vi "MegaAwesome_11_16_12a_OriginDis_JW.vi"() -> ()   [LabVIEW 2011]
uses:
  data/MegaAwesome_States.ctl
  <vilib>/Utility/inputDevices.llb/keyboardAcquire.vi
  <vilib>/Utility/file.llb/Read From Spreadsheet File (string).vi
  <vilib>/Utility/file.llb/Write To Spreadsheet File (string).vi
panel:
  out "Save Next?":bool
  out "Image Center X":i32
  in  "Disable Flag":bool
  out "Index":string
  in  "Slider Min":dbl=5.0
  in  "Slider Max":dbl=5.0
  out "Opj X Axis":string
  out "X Axis Display Type":string
  in  "Index-Sat":dbl=5.0
  in  "Index-Lin":dbl=5.0
  in  "IndexLog-Lin":dbl=5.0
  in  "IndexLog-Sat":dbl=5.0 caption="Num Pts"
  out "Lin Id-Log Used":dbl[](array[numeric])
  out "Lin-Vg Array-Log Used":dbl[](array[numeric])
  out "Save Array":string[][](array[string])
  out "Folder Index":i32 caption="Length"
  out "Sat Id-Used":dbl[](array[numeric])
  out "Sat Vg Array-Used":dbl[](array[numeric])
  out "Vg Array-Log-Used":dbl[](array[numeric])
  out "Sat Id-Log-Used":dbl[](array[numeric])
  out "Lin Id-Used":dbl[](array[numeric])
  out "Lin-Vg Array-Used":dbl[](array[numeric])
  out "Lin Vd":dbl
  out "Recorded Prop":T1
  out "Current State":T2
  in  "Main Tab Control":T3(tab)
  in  "Transfer File":path
  out "Transfer Folder":path
  in  "Transport\nFolder":path caption="Transport Folder"
  out "Transport\nFile":path caption="Transport File"
  in  "Image Folder":path
  out "Image File":path
  out "Fabrication Prop":T4
  out "Distances":i32[](array[numeric])
  in  "Zoom":i32(slide)=-3 scale=-5.0..5.0
  in  "Magnification":i32(ring) items=["5x", "10x", "20x", "50x", "80x"]
  in  "Undo Button":bool
  in  "Remove Button":bool
  in  "Transfer Plots":T5(tab)=enum."Saturation"
  in  "Lin-Trans Slider":dbl(slide) step=1.0 scale=-40.0..40.0 scale format="%#_1p"
  out "Sqrt-Lin":cluster{dbl[], dbl[]}[](graph)
  in  "Sat-Trans Slider":dbl(slide) step=1.0 scale=-40.0..40.0 scale format="%#_1p"
  out "Sqrt-Sat":cluster{dbl[], dbl[]}[](graph)
  out "Raw- Lin":cluster{dbl[], dbl[]}[](graph)
  out "Raw- Sat":cluster{dbl[], dbl[]}[](graph)
  in  "Log Plots":enum32{"Linear", "Saturation", "Transport"}(tab)=enum."Saturation"
  in  "Lin-Log Slider":dbl(slide) step=1.0 scale=-40.0..40.0 scale format="%#_1p"
  out "Lin-Log":cluster{dbl[], dbl[]}[](graph)
  in  "Sat-Log Slider":dbl(slide) step=1.0 scale=-40.0..40.0 scale format="%#_1p"
  out "Sat-Log":cluster{dbl[], dbl[]}[](graph)
  out "Transport":cluster{ext[], ext[]}[](graph)
  out "Transport Name:":string
  in  "Manual Controls":T6
  in  "File Controls":T7
  out "Date Recorded":string="Date Recorded" caption="Measured"
  out "Data Name:":string
  out "Image Name":string
  out "Date Created":string caption="Fabricated"
  in  "Comments:":string
  out "Rec: Length":dbl caption="Length"
  out "Rec: Width":dbl caption="Width"
  out "Rec: Dielectric (d)":dbl caption="Dielectric (d)" format="%#_3g"
  in  "New: Dielectric":dbl
  in  "New: Length":dbl
  in  "New: Width":dbl
  out "Rec: Temp":dbl caption="Sample Temp" format="%.1f"
  in  "New: Temp":dbl format="%.1f"
  out "Image Out":T8(plugin-control)
  in  "Num Pts":i32=5
  in  "Num Pts Log":i32=5 caption="Num Pts"
  out "Recorded Values Cluster":T9
  out "Calculated Values Cluster":T9 caption="Recorded Values Cluster"
  out "Re-Calculated Values Cluster":T9 caption="Recorded Values Cluster"
  in  "Independant Variable:":string(combo)="Length (um):"
  out "Image Preview":T8(plugin-control)
  out "Total Width":i32
  in  "Index Array":i32(ring) caption="Index" items=["4C", "4C", "4C", "4C", "4C", "4C", "4C", "4C", "4C", "4C", "4C", "4C", "4C", "4C", "4C", "4C", "4C", "4C", "4C", "4C", "4C", "4C", "4C", "4C", "4C", "4C", "4C", "4C", "4C", "4C", "4C", "4C", "4C", "4C", "4C", "4C", "4C", "4C", "4C"]
  in  "Room Temp":dbl=294.0 caption="Room Temp (K)"
  out "No Image\n File":path=path "\\\\acad1\\physics/Jurchescu-group/JW-PD/Mega Awesome/Image Not Found.png" caption="No Image File"
  out "Origin Project File":path=path "\\\\acad1\\physics/Jurchescu-group/JW-PD/Group Library/Origin Project Files/DeviceData_8_10_12a_JW.opj"
  out "No Transport\n File":path=path "\\\\acad1\\physics/Jurchescu-group/JW-PD/Mega Awesome/No Transport File.txt" caption="No Transport File"
  in  "Transport Style Controls":T10={"Transport Line Size"=1, "Transport Line Color"=16772608} {"Transport Line Size" items=["Extra Small", "Small", "Medium", "Large", "Extra Large"]}
  out "Application Directory":path
  # "1)  Select the Transfer File that you would like to analyze:"
  # "Transfer Location"
  # "2) What else would you like to view during your analysis?"
  # "Transport Location"
  # "Image Location"
  # "Recorded"
  # "Calculated"
  # "Re-Calculated"
  # "Manual"
  # "um"
  # "V"
  # "V"
  # "V"
  # "Default File Choices"
  # "Default Analysis Values"
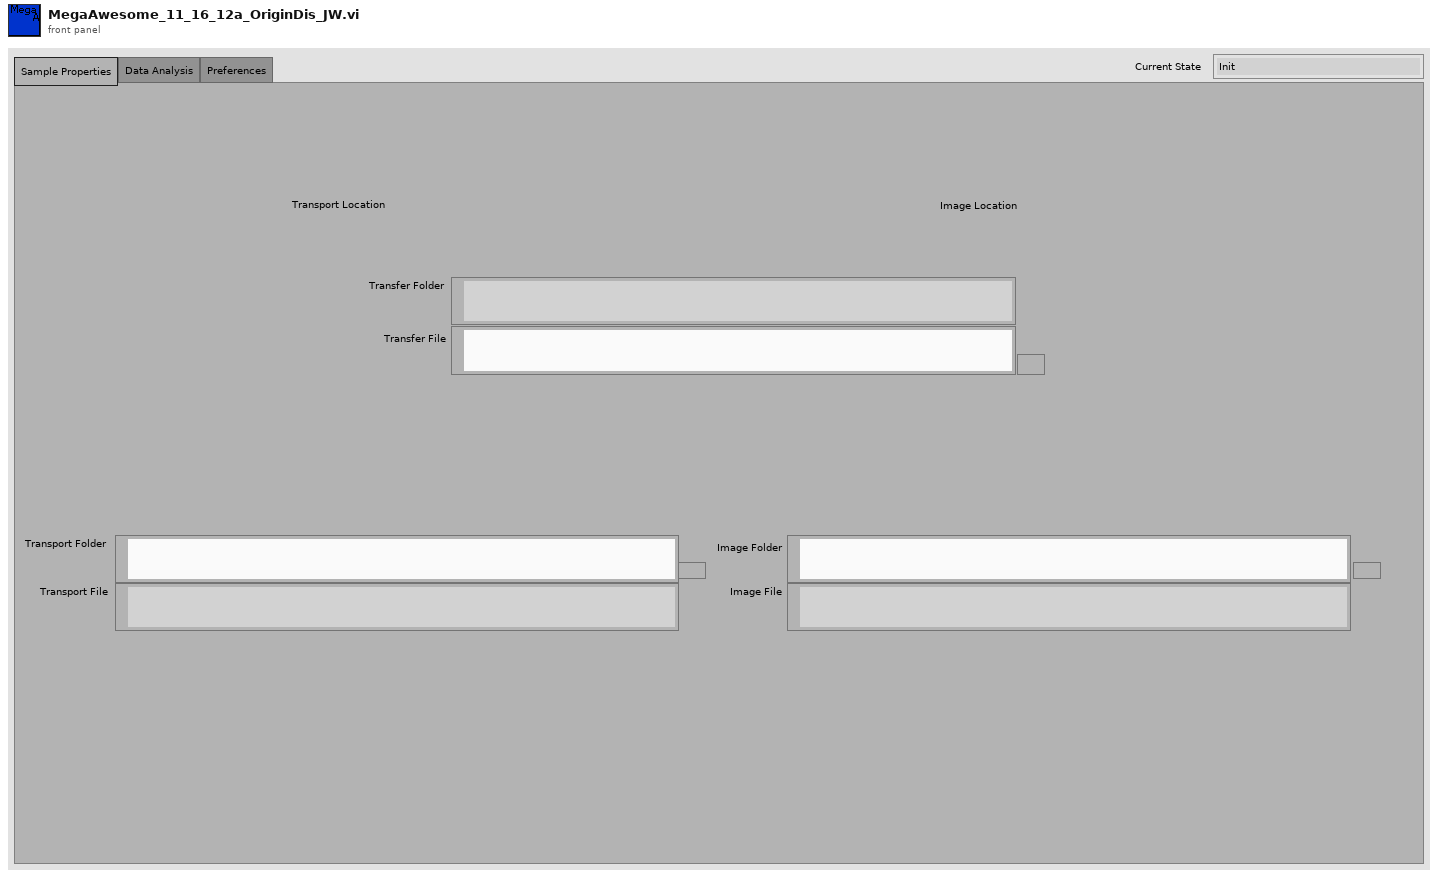
[diagram p1: front panel]
types:
  T1 = cluster{"Date Recorded":string, "Index":string, "Length":dbl, "Width":dbl, "Sample Temp":dbl}
  T2 = typedef "MegaAwesome_States.ctl" = enum16{"Init", "File Missing", "No Event", "Read Data", "Calculated Values", "Re-Calculated Values", "Next File", "Previous File", "Discard File", "Save", "Save Lines", "Export", "Exit"}
  T3 = enum32{"Sample Properties", "Data Analysis", "Preferences"}
  T4 = cluster{"Date Created":string, "Material":string, "Solvent":string, "Concentration":dbl, "Method":string, "Dielectric (nm)":dbl, "Treatment":string, "Comments":string}
  T5 = enum32{"Linear", "Saturation", "Raw-Linear", "Raw-Saturation"}
  T6 = cluster{"Manual-Temp":bool, "Manual-Width":bool, "Manuel-Length":bool, "Manuel-Dielectric":bool, "Manual Comments":bool}
  T7 = cluster{"Previous File":bool, "Discard ":bool, "Save Lines":bool, "Close":bool, "Next File ":bool, "Save":bool, "Save Next":bool, "Export":bool}
  T8 = typedef "IMAQ Image.ctl" = refnum<image>
  T9 = cluster{"Mobility-Sat":dbl, "Moblitity-Lin":dbl, "On/Off":dbl, "Off Current":dbl, "Vt-Sat":dbl, "STS":dbl, "Trap Density-VT":dbl, "Trap Density-STS":dbl}
  T10 = cluster{"Transport Line Size":u16, "Transport Line Color":u32}
  T11 = enum8{"Enabled", "Disabled", "Disabled and Grayed Out"}
  T12 = typedef "LVBoundsTypeDef.ctl" = cluster{"Width":u32, "Height":u32}
  T13 = enum16{"0", "1", "2", "3", "4", "5", "6", "7", "8", "9", "A", "B", "C", "D", "E", "F", "G", "H", "I", "J", "K", "L", "M", "N", "O", "P", "Q", "R", "S", "T", "U", "V", "W", "X", "Y", "Z", "F1", "F2", "F3", "F4", "F5", "F6", "F7", "F8", "F9", "F10", "F11", "F12", "F13", "F14", "F15", "ADD", "BACK", "BACKSLASH", "CAPITAL", "COMMA", "DECIMAL", "DELETE", "DIVIDE", "DOWN", "END", "EQUALS", "ESCAPE", "GRAVE (`)", "HOME", "INSERT", "LBRACKET", "LCONTROL", "LEFT", "L ALT", "LSHIFT", "LWIN", "MINUS", "MULTIPLY", "NEXT", "NUMLOCK", "NUMPAD_0", "NUMPAD_1", "NUMPAD_2", "NUMPAD_3", "NUMPAD_4", "NUMPAD_5", "NUMPAD_6", "NUMPAD_7", "NUMPAD_8", "NUMPAD_9", "PAUSE", "PERIOD", "PRIOR (PG UP)", "RBRACKET", "RCONTROL", "RETURN", "RIGHT", "R ALT", "RSHIFT", "RWIN", "SCROLL", "SEMICOLON", "SLASH", "SPACE", "SUBTRACT", "TAB", "UP", "ENTER (num pad)", "' (quote)"}[]
  T14 = enum16{"0", "1", "2", "3", "4", "5", "6", "7", "8", "9", "A", "B", "C", "D", "E", "F", "G", "H", "I", "J", "K", "L", "M", "N", "O", "P", "Q", "R", "S", "T", "U", "V", "W", "X", "Y", "Z", "F1", "F2", "F3", "F4", "F5", "F6", "F7", "F8", "F9", "F10", "F11", "F12", "F13", "F14", "F15", "ADD", "BACK", "BACKSLASH", "CAPITAL", "COMMA", "DECIMAL", "DELETE", "DIVIDE", "DOWN", "END", "EQUALS", "ESCAPE", "GRAVE (`)", "HOME", "INSERT", "LBRACKET", "LCONTROL", "LEFT", "L ALT", "LSHIFT", "LWIN", "MINUS", "MULTIPLY", "NEXT", "NUMLOCK", "NUMPAD_0", "NUMPAD_1", "NUMPAD_2", "NUMPAD_3", "NUMPAD_4", "NUMPAD_5", "NUMPAD_6", "NUMPAD_7", "NUMPAD_8", "NUMPAD_9", "PAUSE", "PERIOD", "PRIOR (PG UP)", "RBRACKET", "RCONTROL", "RETURN", "RIGHT", "R ALT", "RSHIFT", "RWIN", "SCROLL", "SEMICOLON", "SLASH", "SPACE", "SUBTRACT", "TAB", "UP", "ENTER (num pad)", "' (quote)"}
  T15 = typedef "ROI Descriptor" = cluster{"Global Rectangle":i32[], "Contours":cluster{"ID":enum32{"External", "Internal"}, "Type":u32, "Coordinates":i32[]}[]}
  T16 = cluster{string, sgl, bool, bool, bool, bool, bool, bool, i32}
  T17 = cluster{i32, cluster{string, sgl, bool, bool, bool, bool, bool, bool, i32}, i32, i32}
  T18 = cluster{"Global Rectangle":i32[], "Contours":cluster{"Contour Type":u32, "ROI Type":u32, "Points":i32[]}[]}
  T19 = cluster{"Contour Type":u32, "ROI Type":u32, "Points":i32[]}[]
  T20 = cluster{"[0]":cluster{dbl[], dbl[]}, "[1]":cluster{dbl[], dbl[]}, "[2]":cluster{dbl[], dbl[]}, "[3]":cluster{dbl[], dbl[]}, "[4]":cluster{dbl[], dbl[]}, "[5]":cluster{dbl[], dbl[]}, "[6]":cluster{dbl[], dbl[]}, "[7]":cluster{dbl[], dbl[]}, "[8]":cluster{dbl[], dbl[]}}
  T21 = cluster{i32[], cluster{"Contour Type":u32, "ROI Type":u32, "Points":i32[]}[]}
  T22 = cluster{"Contour Type":u32, "ROI Type":u32, "Points":i32[]}
  T23 = cluster{"Points[0]":i32, "Points[1]":i32, "Points[2]":i32, "Points[3]":i32, "Points[4]":i32, "Points[5]":i32, "Points[6]":i32, "Points[7]":i32, "Points[8]":i32}
  T24 = cluster{"Sat Vg Used":dbl[], "Sat Sqrt(Id) Used ":dbl[], "Lin Vg Used":dbl[], "Lin Sqrt(Id) Used":dbl[], "Index-Lin":dbl, "Index-Sat":dbl}
  T25 = cluster{"Raw Sat":cluster{dbl[], dbl[]}[], "Sqrt Sat":cluster{dbl[], dbl[]}[], "Log Sat":cluster{dbl[], dbl[]}[], "Raw Lin":cluster{dbl[], dbl[]}[], "Sqrt Lin":cluster{dbl[], dbl[]}[], "Log Lin":cluster{dbl[], dbl[]}[]}
  T26 = cluster{"Mobility-Sat":dbl, "Vt-Sat":dbl, "Mobility-Lin":dbl, "Vt-Lin":dbl, "Off I-Sat":dbl, "On/Off I-Sat":dbl}
  T27 = cluster{"Sat Vg Used":dbl[], "Sat Log(Id) Used":dbl[], "Lin Vg Used":dbl[], "Lin Log(Id) Used":dbl[], "STS Index-Sat":dbl, "STS Index-Lin":dbl}
  T28 = cluster{"Independant  Variable Indicator":string, "Parameter String Indicator":string}
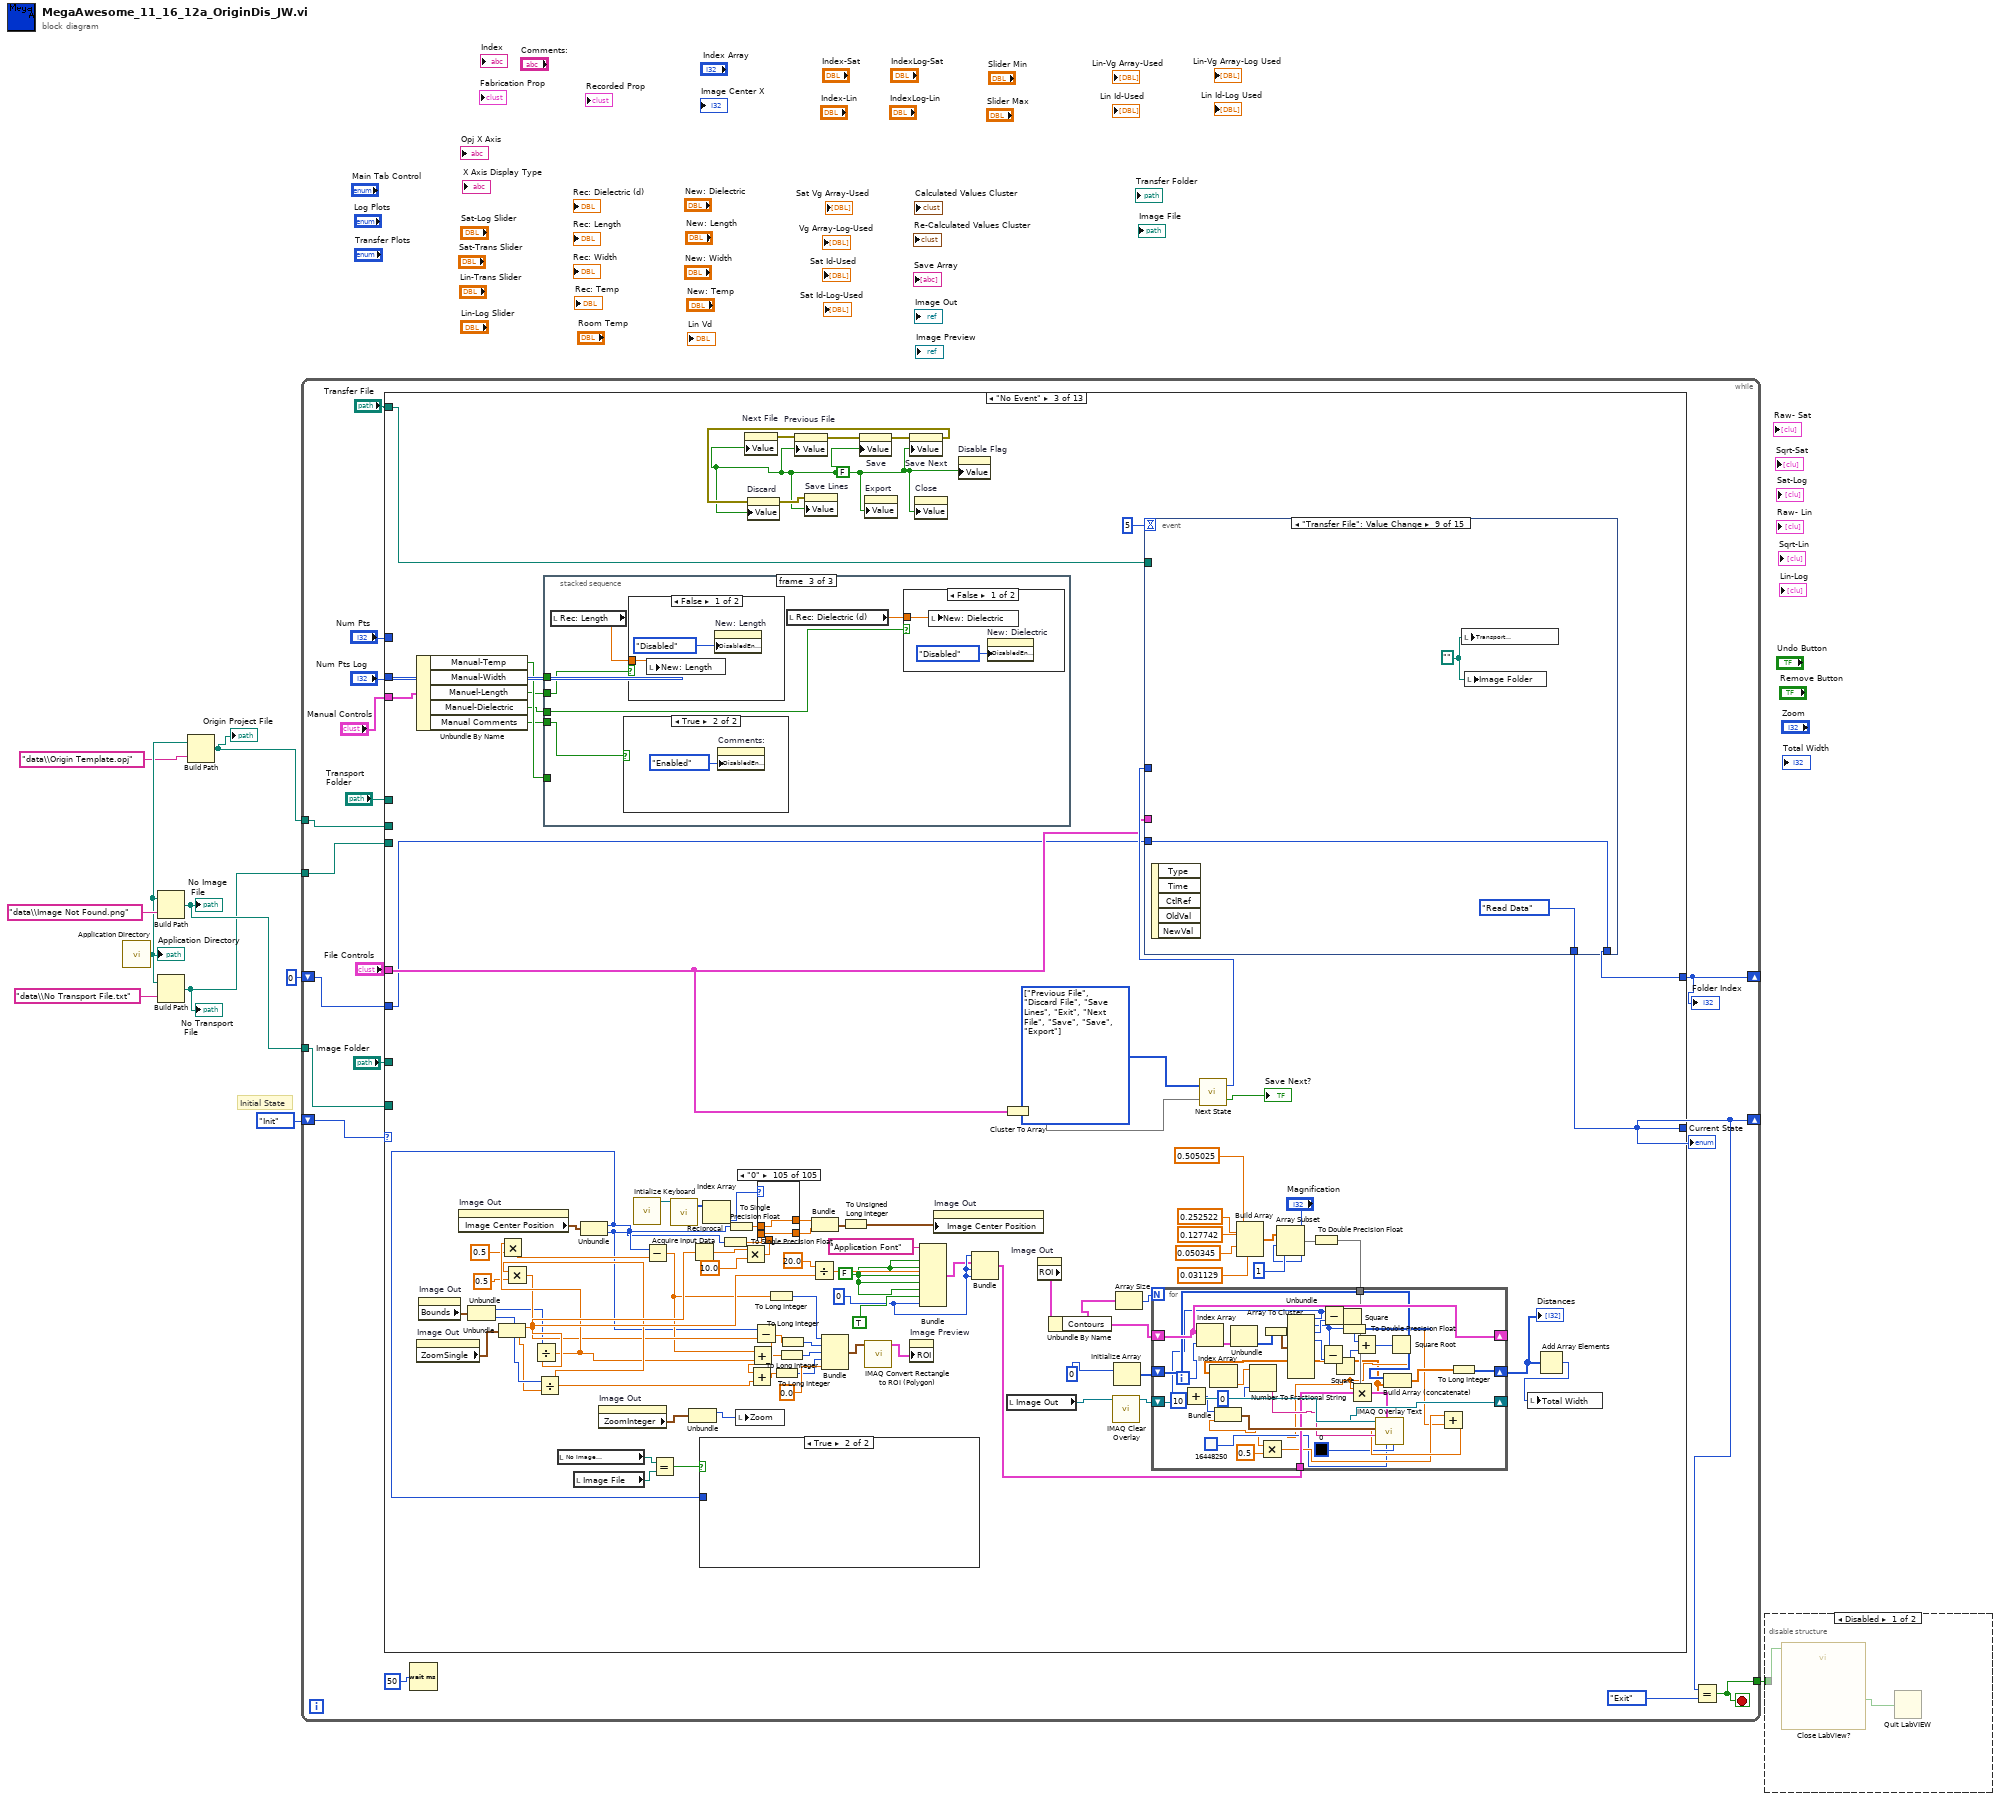
[diagram p0: block diagram]
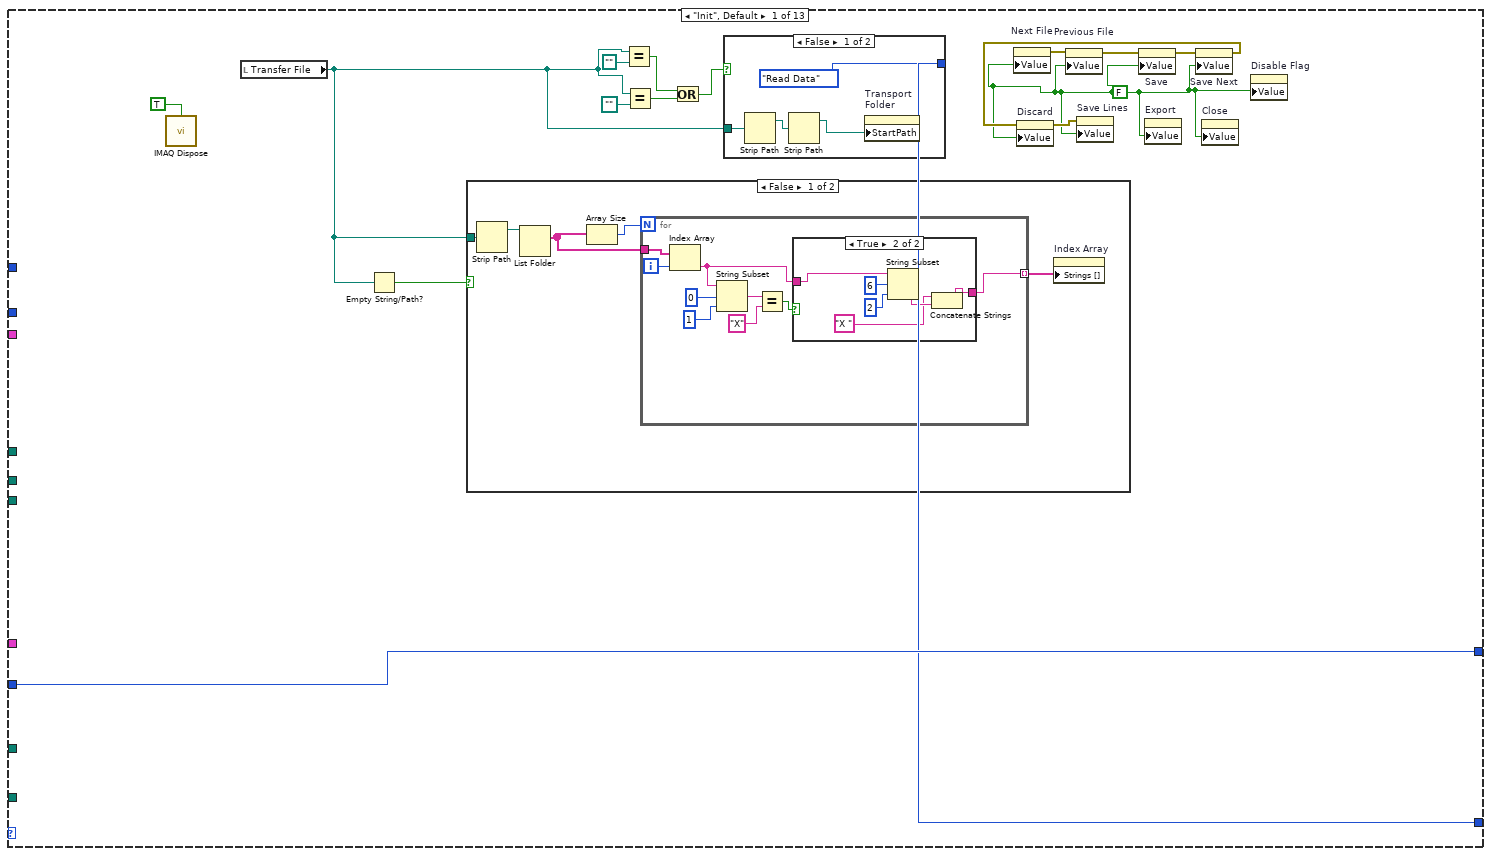
[diagram p3: hidden frame]
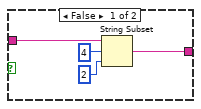
[diagram p4: hidden frame]
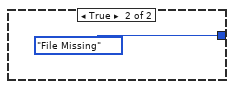
[diagram p6: hidden frame]
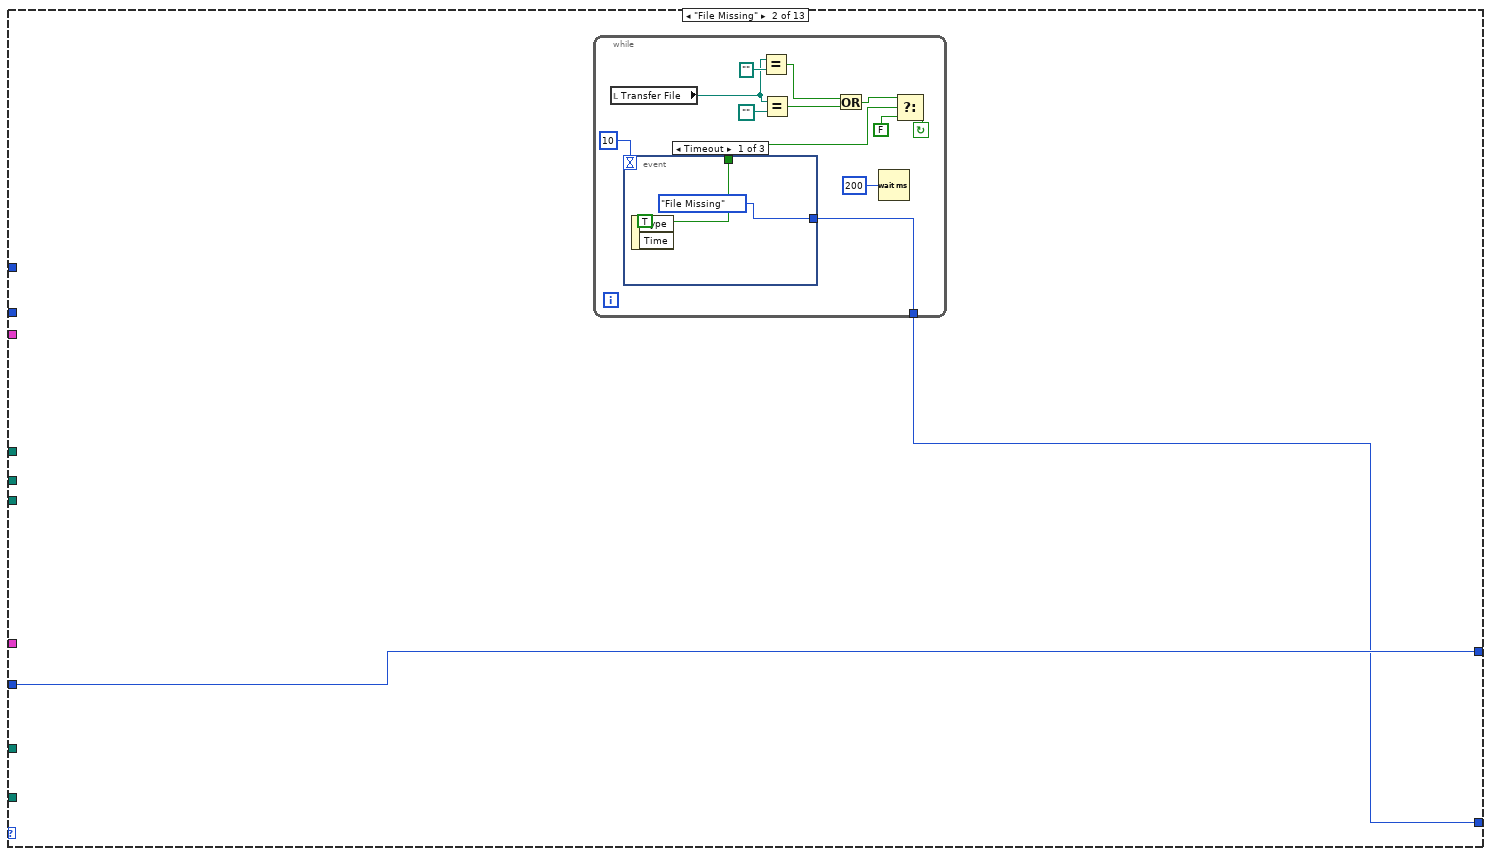
[diagram p7: hidden frame]
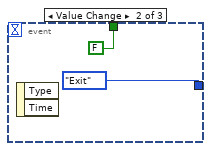
[diagram p8: hidden frame]
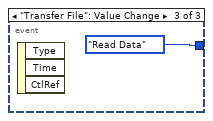
[diagram p9: hidden frame]
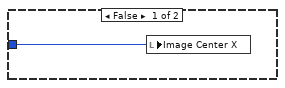
[diagram p10: hidden frame]
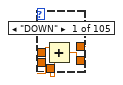
[diagram p11: hidden frame]
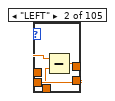
[diagram p12: hidden frame]
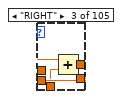
[diagram p13: hidden frame]
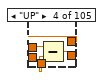
[diagram p14: hidden frame]
diagram:
  # "Initial State"
  n1 = call <vilib>:"Application Directory.vi"() -> ("Application Directory"=w3:path)
  "Application Directory" <- w3
  n2 = Build Path(base path=w3, name or relative path="data\\Image Not Found.png") -> (appended path=w6:path)
  "No Image\n File" <- w6
  n3 = Build Path(base path=w3, name or relative path="data\\No Transport File.txt") -> (appended path=w5:path)
  "No Transport\n File" <- w5
  n4 = Build Path(base path=w3, name or relative path="data\\Origin Template.opj") -> (appended path=w4:path)
  "Origin Project File" <- w4
  n5 = while {
    shift-right: [w11] -> _
    shift-left: MegaAwesome_States."Init" -> [w13]
    shift-right: [w21] -> _
    shift-left: 0 -> [w22]
    tunnel: w6 -> [w18]
    tunnel: w5 -> [w16]
    tunnel: w4 -> [w15]
    tunnel: [w14] -> w1
    stop <- w14 stop-if-true
    n6 = case shown="\"No Event\"" w13 {
      tunnel: [w29 w73 w174 MegaAwesome_States."Calculated Values" MegaAwesome_States."Re-Calculated Values" MegaAwesome_States."No Event" MegaAwesome_States."Read Data" MegaAwesome_States."Read Data" MegaAwesome_States."Init" w828 MegaAwesome_States."Exit" MegaAwesome_States."No Event" MegaAwesome_States."No Event"] -> w11
      tunnel: "Transfer File" -> [_ _ w166 w627 w675 _ w776 w787 w814 w833 _ _ _]
      tunnel: "Num Pts" -> [_ _ _ _ w710 _ _ _ _ _ _ _ _]
      tunnel: "Num Pts Log" -> [_ _ _ _ w709 _ _ _ _ _ _ _ _]
      tunnel: "Image Folder" -> [_ _ _ _ w706 _ _ _ _ _ _ w1340 _]
      tunnel: w18 -> [_ _ _ _ w705 _ _ _ _ _ _ _ _]
      tunnel: [w38 w74 w167 w632 w704 w736 w762 w785 w810 w834 w1326 w1350 w1356] -> w21
      tunnel: w22 -> [w38 w74 w108 w630 w704 w736 w763 w786 _ w834 w1326 w1350 w1356]
      tunnel: "Manual Controls" -> [_ _ w176 _ _ _ _ _ _ w832 _ _ _]
      tunnel: "File Controls" -> [_ _ w164 _ _ _ _ _ _ _ _ _ _]
      tunnel: "Transport\nFolder" -> [_ _ _ _ w671 _ _ _ _ _ _ _ _]
      tunnel: w16 -> [_ _ _ _ w670 _ _ _ _ _ _ _ _]
      tunnel: w15 -> [_ _ _ _ _ _ _ _ _ _ _ _ w1355]
      frame "Init", Default {
        w30 = FALSE
        n7 = call "IMAQ Dispose"("All Images? (No)"=TRUE) -> ()  [unwired: 5 in, 1 out]
        n8 = local read "Transfer File"() -> (w28:path)
        n9 = Empty String/Path?(string/path=w28) -> (empty?=w37:bool)
        n10 = case shown="False" w37 {
          tunnel: w28 -> [w45 _]
          frame False {
            n11 = Strip Path(path=w45) -> (stripped path=w47:path)  [unwired: 1 out]
            n12 = List Folder(path=w47) -> (filenames=w46:string[])  [unwired: 3 in, 3 out]
            n13 = Array Size(array=w46) -> (size(s)=w48:i32)
            n14 = for {
              N: w48 -> [_]
              tunnel: w46 -> [w57]
              tunnel: [w55] -> w44 mode=indexing
              i -> [w56]
              n15 = Index Array(array=w57, index=w56) -> (element=w54:string)
              n16 = String Subset(string=w54, offset (0)=0, length (rest)=1) -> (substring=w51:string)
              n17 = Equal?(x=w51, y="X") -> (x = y?=w50:bool)
              n18 = case shown="True" w50 {
                tunnel: w54 -> [w61 w65]
                tunnel: [w58 w64] -> w55
                frame False {
                  n19 = String Subset(string=w61, offset (0)=4, length (rest)=2) -> (substring=w58:string)
                }
                frame True {
                  n20 = String Subset(string=w65, offset (0)=6, length (rest)=2) -> (substring=w63:string)
                  n21 = Concatenate Strings("X ", w63) -> (w64:string)
                }
              }
            }
            n22 = property on="Index Array" class="Ring (strict)"("Strings []"=w44) -> ()  [unwired: 2 in, 2 out]
          }
          frame True {
          }
        }
        n23 = Equal?(x=w28, y=path "") -> (x = y?=w41:bool)
        n24 = Equal?(x=w28, y=path "") -> (x = y?=w40:bool)
        n25 = Or(x=w41, y=w40) -> (x .or. y?=w43:bool)
        n26 = case shown="False" w43 {
          tunnel: [MegaAwesome_States."Read Data" MegaAwesome_States."File Missing"] -> w29
          tunnel: w28 -> [w70 _]
          frame False {
            n27 = Strip Path(path=w70) -> (stripped path=w69:path)  [unwired: 1 out]
            n28 = Strip Path(path=w69) -> (stripped path=w68:path)  [unwired: 1 out]
            n29 = property on="Transport\nFolder" class="Path"("StartPath"=w68) -> ()  [unwired: 2 in, 2 out]
          }
          frame True {
          }
        }
        n30 = property on="Next File" class="Bool (strict)"("Value"=w30) -> (error out=w35:errorcluster)  [unwired: 2 in, 1 out]
        n31 = property on="Previous File" class="Bool (strict)"(error in=w35, "Value"=w30) -> (error out=w34:errorcluster)  [unwired: 1 in, 1 out]
        n32 = property on="Save" class="Bool (strict)"(error in=w34, "Value"=w30) -> (error out=w33:errorcluster)  [unwired: 1 in, 1 out]
        n33 = property on="Export" class="Bool (strict)"("Value"=w30) -> ()  [unwired: 2 in, 2 out]
        n34 = property on="Save Next" class="Bool (strict)"(error in=w33, "Value"=w30) -> (error out=w32:errorcluster)  [unwired: 1 in, 1 out]
        n35 = property on="Discard" class="Bool (strict)"(error in=w32, "Value"=w30) -> (error out=w31:errorcluster)  [unwired: 1 in, 1 out]
        n36 = property on="Save Lines" class="Bool (strict)"(error in=w31, "Value"=w30) -> ()  [unwired: 1 in, 2 out]
        n37 = property on="Close" class="Bool (strict)"("Value"=w30) -> ()  [unwired: 2 in, 2 out]
        n38 = property on="Disable Flag" class="Bool (strict)"("Value"=w30) -> ()  [unwired: 2 in, 2 out]
      }
      frame "File Missing" {
        n39 = while {
          tunnel: [w81] -> w73
          stop <- w77 continue-if-true
          n40 = local read "Transfer File"() -> (w82:path)
          n41 = event shown="[0] Timeout" {
            selector: _ -> [_ _ _]
            dyn-events: _ -> [_ _ _]
            timeout: 10 -> [_ _ _]
            tunnel: [MegaAwesome_States."File Missing" MegaAwesome_States."Exit" MegaAwesome_States."Read Data"] -> w81
            tunnel: [TRUE FALSE _] -> w80
            event Timeout {
              n42 = event-data() -> ()  [unwired: 1 in, 2 out]
            }
            event "File Controls.Close": Value Change {
              n43 = event-data() -> ()  [unwired: 1 in, 2 out]
            }
            event "Transfer File": Value Change {
              n44 = event-data() -> ()  [unwired: 1 in, 3 out]
            }
          }
          n45 = Equal?(x=w82, y=path "") -> (x = y?=w84:bool)
          n46 = Equal?(x=w82, y=path "") -> (x = y?=w85:bool)
          n47 = Or(x=w84, y=w85) -> (x .or. y?=w79:bool)
          n48 = Wait (ms)(milliseconds to wait=u32 200) -> ()  [unwired: 1 out]
          n49 = Select(t=w79, s=w80, f=FALSE) -> (s? t:f=w77:bool)
        }
      }
      frame "No Event" {
        w155 = FALSE
        w157 = 0
        w165 = FALSE
        w183 = T2[] [enum."Previous File", enum."Discard File", enum."Save Lines", enum."Exit", enum."Next File", enum."Save", enum."Save", enum."Export"] items=["Init", "File Missing", "No Event", "Read Data", "Calculated Values", "Re-Calculated Values", "Next File", "Previous File", "Discard File", "Save", "Save Lines", "Export", "Exit"]
        n50 = Unbundle By Name(w176) -> ("Manual-Temp"=w181:bool, "Manual-Width"=w180:bool, "Manuel-Length"=w179:bool, "Manuel-Dielectric"=w178:bool, "Manual Comments"=w177:bool)
        n51 = property on="Image Out" class="ImageControl"() -> ("ZoomSingle"=w144:cluster{"X":sgl, "Y":sgl})  [unwired: 2 in, 2 out]
        n52 = property on="Image Out" class="ImageControl"() -> ("Bounds"=w143:T12)  [unwired: 2 in, 2 out]
        n53 = property on="Image Out" class="ImageControl"() -> ("Image Center Position"=w140:cluster{"X":u32, "Y":u32})  [unwired: 2 in, 2 out]
        n54 = Unbundle(w143) -> ("Width"=w146:u32, "Height"=w147:u32)
        n55 = Unbundle(w144) -> ("X"=w161:sgl, "Y"=w145:sgl)
        n56 = Divide(x=w146, y=w161) -> (x/y=w152:sgl)
        n57 = Multiply(x=w152, y=sgl 0.5) -> (x*y=w150:sgl)
        n58 = Divide(x=w147, y=w145) -> (x/y=w153:sgl)
        n59 = Multiply(x=w153, y=sgl 0.5) -> (x*y=w151:sgl)
        n60 = stacked-sequence {
          tunnel: w181 -> [w585 _ _]
          tunnel: w180 -> [_ w599 _]
          tunnel: w179 -> [_ _ w612]
          tunnel: w178 -> [_ _ w610]
          tunnel: w177 -> [_ _ w609]
          frame #0 {
            n61 = local read "Rec: Temp"() -> (w584:dbl)
            n62 = case shown="True" w585 {
              tunnel: w584 -> [w590 _]
              frame False {
                n63 = local read "Rec: Temp"() -> (w588:dbl)
                n64 = property on="New: Temp" class="DigNum (strict)"("DisabledEnum"=T11."Disabled" ("Disabled")) -> ()  [unwired: 2 in, 2 out]
                n65 = Equal To 0?(x=w588) -> (x = 0?=w589:bool)
                n66 = local write "New: Temp"(w590) -> ()
                n67 = case shown="True" w589 {
                  tunnel: [w591 w592] -> w586
                  tunnel: w588 -> [w591 _]
                  frame False {
                  }
                  frame True {
                    n68 = local read "Room Temp"() -> (w592:dbl)
                  }
                }
                n69 = local write "Rec: Temp"(w586) -> ()
                n70 = local write "New: Temp"(w586) -> ()
              }
              frame True {
                n71 = property on="New: Temp" class="DigNum (strict)"("DisabledEnum"=T11."Enabled" ("Disabled")) -> ()  [unwired: 2 in, 2 out]
              }
            }
          }
          frame #1 {
            n72 = local read "New: Width"() -> (w600:dbl)
            n73 = local read "Total Width"() -> (w596:i32)
            n74 = case shown="False" w599 {
              frame False {
                n75 = property on="New: Width" class="DigNum (strict)"("DisabledEnum"=T11."Disabled" ("Disabled")) -> ()  [unwired: 2 in, 2 out]
              }
              frame True {
                n76 = property on="New: Width" class="DigNum (strict)"("DisabledEnum"=T11."Enabled" ("Disabled")) -> ()  [unwired: 2 in, 2 out]
              }
            }
            n77 = Not(x=w599) -> (.not. x?=w594:bool)
            n78 = Not Equal?(x=w596, y=w600) -> (x != y?=w595:bool)
            n79 = Equal To 0?(x=w596) -> (x = 0?=w598:bool)
            n80 = And(x=w594, y=w598) -> (x .and. y?=w597:bool)
            n81 = case shown="False" w597 {
              tunnel: w596 -> [w604 _]
              tunnel: w595 -> [w603 _]
              tunnel: w594 -> [w602 _]
              frame False {
                n82 = And(x=w602, y=w603) -> (x .and. y?=w601:bool)
                n83 = case shown="True" w601 {
                  tunnel: w604 -> [_ w605]
                  frame False {
                  }
                  frame True {
                    n84 = property on="New: Width" class="DigNum (strict)"("Val(Sgnl)"=w605) -> ()  [unwired: 2 in, 2 out]
                  }
                }
              }
              frame True {
                n85 = local read "Rec: Width"() -> (w606:dbl)
                n86 = local write "New: Width"(w606) -> ()
              }
            }
          }
          frame #2 {
            n87 = local read "Rec: Length"() -> (w613:dbl)
            n88 = case shown="True" w609 {
              frame False {
                n89 = property on="Comments:" class="Str"("DisabledEnum"=T11."Disabled" ("Disabled")) -> ()  [unwired: 2 in, 2 out]
              }
              frame True {
                n90 = property on="Comments:" class="Str"("DisabledEnum"=T11."Enabled" ("Disabled")) -> ()  [unwired: 2 in, 2 out]
              }
            }
            n91 = case shown="False" w612 {
              tunnel: w613 -> [w620 _]
              frame False {
                n92 = local write "New: Length"(w620) -> ()
                n93 = property on="New: Length" class="DigNum (strict)"("DisabledEnum"=T11."Disabled" ("Disabled")) -> ()  [unwired: 2 in, 2 out]
              }
              frame True {
                n94 = property on="New: Length" class="DigNum (strict)"("DisabledEnum"=T11."Enabled" ("Disabled")) -> ()  [unwired: 2 in, 2 out]
              }
            }
            n95 = local read "Rec: Dielectric (d)"() -> (w611:dbl)
            n96 = case shown="False" w610 {
              tunnel: w611 -> [w617 _]
              frame False {
                n97 = local write "New: Dielectric"(w617) -> ()
                n98 = property on="New: Dielectric" class="DigNum (strict)"("DisabledEnum"=T11."Disabled" ("Disabled")) -> ()  [unwired: 2 in, 2 out]
              }
              frame True {
                n99 = property on="New: Dielectric" class="DigNum (strict)"("DisabledEnum"=T11."Enabled" ("Disabled")) -> ()  [unwired: 2 in, 2 out]
              }
            }
          }
        }
        n100 = local read "No Image\n File"() -> (w114:path)
        n101 = local read "Image File"() -> (w113:path)
        n102 = Unbundle(w140) -> ("X"=w94:u32, "Y"=w92:u32)
        n103 = property on="Image Out" class="ImageControl"() -> ("ZoomInteger"=w117:cluster{"X":i32, "Y":i32})  [unwired: 2 in, 2 out]
        n104 = call <vilib>:"Intialize Keyboard.vi"() -> ("device ID"=w138:refnum<k1>)  [unwired: 10 in, 1 out]
        n105 = Subtract(x=w94, y=w150) -> (x-y=w102:sgl)
        n106 = Equal?(x=w114, y=w113) -> (x = y?=w112:bool)
        n107 = call-poly <vilib>:"Acquire Input Data.vi"("device ID"=w138) -> ("keys pressed"=w139:T13)  [unwired: 16 in, 2 out]
        n108 = Unbundle(w117) -> ("X"=w116:i32)  [unwired: 1 out]
        n109 = Reciprocal(x=w161) -> (1/x=w162:sgl)
        n110 = case shown="True" w112 {
          tunnel: w94 -> [w184 _]
          frame False {
            n111 = local write "Image Center X"(w184) -> ()
          }
          frame True {
          }
        }
        n112 = Index Array(array=w139) -> (element=w96:T14)  [unwired: 1 in]
        n113 = To Single Precision Float(number=w92) -> (single precision float=w93:sgl)
        n114 = To Single Precision Float(number=w94) -> (single precision float=w95:sgl)
        n115 = local write "Zoom"(w116) -> ()
        n116 = Multiply(x=w162, y=sgl 10.0) -> (x*y=w160:sgl)
        n117 = property on="Next File" class="Bool (strict)"("Value"=w165) -> (error out=w172:errorcluster)  [unwired: 2 in, 1 out]
        n118 = Add(x=w102, y=w152) -> (x+y=w100:sgl)
        n119 = Subtract(x=w92, y=w151) -> (x-y=w104:sgl)
        n120 = Add(x=w104, y=w153) -> (x+y=w98:sgl)
        n121 = case shown="\"0\"" w96 {
          tunnel: w95 -> [w221 w227 w231 w233 w237 w239 w241 w243 w245 w247 w249 w251 w253 w255 w257 w259 w261 w263 w265 w267 w269 w271 w273 w275 w277 w279 w281 w283 w285 w287 w289 w291 w293 w295 w297 w299 w301 w303 w305 w307 w309 w311 w313 w315 w317 w319 w321 w323 w325 w327 w329 w331 w333 w335 w337 w339 w341 w343 w345 w347 w349 w351 w353 w355 w357 w359 w361 w363 w365 w367 w369 w371 w373 w375 w377 w379 w381 w383 w385 w387 w389 w391 w393 w395 w397 w399 w401 w403 w405 w407 w409 w411 w413 w415 w417 w419 w421 w423 w425 w427 w429 w431 w433 w435 w437]
          tunnel: [w221 w226 w230 w233 w237 w239 w241 w243 w245 w247 w249 w251 w253 w255 w257 w259 w261 w263 w265 w267 w269 w271 w273 w275 w277 w279 w281 w283 w285 w287 w289 w291 w293 w295 w297 w299 w301 w303 w305 w307 w309 w311 w313 w315 w317 w319 w321 w323 w325 w327 w329 w331 w333 w335 w337 w339 w341 w343 w345 w347 w349 w351 w353 w355 w357 w359 w361 w363 w365 w367 w369 w371 w373 w375 w377 w379 w381 w383 w385 w387 w389 w391 w393 w395 w397 w399 w401 w403 w405 w407 w409 w411 w413 w415 w417 w419 w421 w423 w425 w427 w429 w431 w433 w435 w437] -> w136
          tunnel: w93 -> [w223 w225 w229 w235 w236 w238 w240 w242 w244 w246 w248 w250 w252 w254 w256 w258 w260 w262 w264 w266 w268 w270 w272 w274 w276 w278 w280 w282 w284 w286 w288 w290 w292 w294 w296 w298 w300 w302 w304 w306 w308 w310 w312 w314 w316 w318 w320 w322 w324 w326 w328 w330 w332 w334 w336 w338 w340 w342 w344 w346 w348 w350 w352 w354 w356 w358 w360 w362 w364 w366 w368 w370 w372 w374 w376 w378 w380 w382 w384 w386 w388 w390 w392 w394 w396 w398 w400 w402 w404 w406 w408 w410 w412 w414 w416 w418 w420 w422 w424 w426 w428 w430 w432 w434 w436]
          tunnel: [w222 w225 w229 w234 w236 w238 w240 w242 w244 w246 w248 w250 w252 w254 w256 w258 w260 w262 w264 w266 w268 w270 w272 w274 w276 w278 w280 w282 w284 w286 w288 w290 w292 w294 w296 w298 w300 w302 w304 w306 w308 w310 w312 w314 w316 w318 w320 w322 w324 w326 w328 w330 w332 w334 w336 w338 w340 w342 w344 w346 w348 w350 w352 w354 w356 w358 w360 w362 w364 w366 w368 w370 w372 w374 w376 w378 w380 w382 w384 w386 w388 w390 w392 w394 w396 w398 w400 w402 w404 w406 w408 w410 w412 w414 w416 w418 w420 w422 w424 w426 w428 w430 w432 w434 w436] -> w137
          tunnel: w160 -> [w220 w224 w228 w232 _ _ _ _ _ _ _ _ _ _ _ _ _ _ _ _ _ _ _ _ _ _ _ _ _ _ _ _ _ _ _ _ _ _ _ _ _ _ _ _ _ _ _ _ _ _ _ _ _ _ _ _ _ _ _ _ _ _ _ _ _ _ _ _ _ _ _ _ _ _ _ _ _ _ _ _ _ _ _ _ _ _ _ _ _ _ _ _ _ _ _ _ _ _ _ _ _ _ _ _ _]
          frame "DOWN" {
            n122 = Add(x=w223, y=w220) -> (x+y=w222:sgl)
          }
          frame "LEFT" {
            n123 = Subtract(x=w227, y=w224) -> (x-y=w226:sgl)
          }
          frame "RIGHT" {
            n124 = Add(x=w231, y=w228) -> (x+y=w230:sgl)
          }
          frame "UP" {
            n125 = Subtract(x=w235, y=w232) -> (x-y=w234:sgl)
          }
          frame "ENTER (num pad)" {
          }
          frame "' (quote)" {
          }
          frame "END" {
          }
          frame "EQUALS" {
          }
          frame "ESCAPE" {
          }
          frame "GRAVE (`)" {
          }
          frame "HOME" {
          }
          frame "INSERT" {
          }
          frame "LBRACKET" {
          }
          frame "LCONTROL" {
          }
          frame "L ALT" {
          }
          frame "LSHIFT" {
          }
          frame "LWIN" {
          }
          frame "MINUS" {
          }
          frame "MULTIPLY" {
          }
          frame "NEXT" {
          }
          frame "NUMLOCK" {
          }
          frame "NUMPAD_0" {
          }
          frame "NUMPAD_1" {
          }
          frame "NUMPAD_2" {
          }
          frame "NUMPAD_3" {
          }
          frame "NUMPAD_4" {
          }
          frame "NUMPAD_5" {
          }
          frame "NUMPAD_6" {
          }
          frame "NUMPAD_7" {
          }
          frame "NUMPAD_8" {
          }
          frame "NUMPAD_9" {
          }
          frame "PAUSE" {
          }
          frame "PERIOD" {
          }
          frame "PRIOR (PG UP)" {
          }
          frame "RBRACKET" {
          }
          frame "RCONTROL" {
          }
          frame "RETURN" {
          }
          frame "R ALT" {
          }
          frame "RSHIFT" {
          }
          frame "RWIN" {
          }
          frame "SCROLL" {
          }
          frame "SEMICOLON" {
          }
          frame "SLASH" {
          }
          frame "SPACE" {
          }
          frame "SUBTRACT" {
          }
          frame "TAB" {
          }
          frame "DIVIDE" {
          }
          frame "DELETE" {
          }
          frame "DECIMAL" {
          }
          frame "COMMA" {
          }
          frame "CAPITAL" {
          }
          frame "BACKSLASH" {
          }
          frame "BACK" {
          }
          frame "ADD" {
          }
          frame "F15" {
          }
          frame "F14" {
          }
          frame "F13" {
          }
          frame "F12" {
          }
          frame "F11" {
          }
          frame "F10" {
          }
          frame "F9" {
          }
          frame "F8" {
          }
          frame "F7" {
          }
          frame "F6" {
          }
          frame "F5" {
          }
          frame "F4" {
          }
          frame "F3" {
          }
          frame "F2" {
          }
          frame "F1" {
          }
          frame "Z" {
          }
          frame "Y" {
          }
          frame "X" {
          }
          frame "W" {
          }
          frame "V" {
          }
          frame "U" {
          }
          frame "T" {
          }
          frame "S" {
          }
          frame "R" {
          }
          frame "Q" {
          }
          frame "P" {
          }
          frame "O" {
          }
          frame "N" {
          }
          frame "M" {
          }
          frame "L" {
          }
          frame "K" {
          }
          frame "J" {
          }
          frame "I" {
          }
          frame "H" {
          }
          frame "G" {
          }
          frame "F" {
          }
          frame "E" {
          }
          frame "D" {
          }
          frame "C" {
          }
          frame "B" {
          }
          frame "A" {
          }
          frame "9" {
          }
          frame "8" {
          }
          frame "7" {
          }
          frame "6" {
          }
          frame "5" {
          }
          frame "4" {
          }
          frame "3" {
          }
          frame "2" {
          }
          frame "1" {
          }
          frame "0" {
          }
        }
        n126 = To Long Integer(number=w102) -> (32bit integer=w101:i32)
        n127 = To Long Integer(number=w98) -> (32bit integer=w97:i32)
        n128 = To Long Integer(number=w100) -> (32bit integer=w99:i32)
        n129 = To Long Integer(number=w104) -> (32bit integer=w103:i32)
        n130 = property on="Previous File" class="Bool (strict)"(error in=w172, "Value"=w165) -> (error out=w171:errorcluster)  [unwired: 1 in, 1 out]
        n131 = Divide(x=sgl 20.0, y=w161) -> (x/y=w159:sgl)
        n132 = Bundle(w136, w137) -> (w107:cluster{sgl, sgl})  [unwired: 1 in]
        n133 = Bundle(w101, w103, w99, w97, 0.0) -> (w105:cluster{i32, i32, i32, i32, dbl})  [unwired: 1 in]
        n134 = To Unsigned Long Integer(number=w107) -> (unsigned 32bit integer=w106:cluster{u32, u32})
        n135 = property on="Save" class="Bool (strict)"(error in=w171, "Value"=w165) -> (error out=w170:errorcluster)  [unwired: 1 in, 1 out]
        n136 = property on="Export" class="Bool (strict)"("Value"=w165) -> ()  [unwired: 2 in, 2 out]
        n137 = call "IMAQ Convert Rectangle to ROI (Polygon)"("Rectangle"=w105) -> ("ROI Descriptor"=w142:T15)  [unwired: 7 in, 2 out]
        n138 = property on="Save Next" class="Bool (strict)"(error in=w170, "Value"=w165) -> (error out=w169:errorcluster)  [unwired: 1 in, 1 out]
        n139 = property on="Discard" class="Bool (strict)"(error in=w169, "Value"=w165) -> (error out=w168:errorcluster)  [unwired: 1 in, 1 out]
        n140 = property on="Save Lines" class="Bool (strict)"(error in=w168, "Value"=w165) -> ()  [unwired: 1 in, 2 out]
        n141 = property on="Image Preview" class="ImageControl"("ROI"=w142) -> ()  [unwired: 2 in, 2 out]
        n142 = property on="Close" class="Bool (strict)"("Value"=w165) -> ()  [unwired: 2 in, 2 out]
        n143 = Bundle("Application Font", w159, w155, w155, w155, w155, w155, TRUE, w157) -> (w154:T16)  [unwired: 1 in]
        n144 = property on="Image Out" class="ImageControl"("Image Center Position"=w106) -> ()  [unwired: 2 in, 2 out]
        n145 = property on="Disable Flag" class="Bool (strict)"("Value"=w165) -> ()  [unwired: 2 in, 2 out]
        n146 = Bundle(w157, w154, w157, w157) -> (w119:T17)  [unwired: 1 in]
        n147 = Cluster To Array(cluster=w164) -> (array=w182:bool[])
        n148 = local read "Image Out"() -> (w118:T8)
        n149 = property on="Image Out" class="ImageControl"() -> ("ROI"=w121:T18)  [unwired: 2 in, 2 out]
        n150 = Unbundle By Name(w121) -> ("Contours"=w122:T19)
        n151 = call "IMAQ Clear Overlay"("Image"=w118) -> ("Image Out"=w135:T8)  [unwired: 9 in, 1 out]
        n152 = Initialize Array(0) -> (w124:i32[])  [unwired: 1 in]
        n153 = Array Size(array=w122) -> (size(s)=w123:i32)
        n154 = call "Next State.vi"("Buttons []"=w182, "States []"=w183) -> ("Save Next?"=→"Save Next?":bool, "Enum"=w175:T2)
        n155 = event shown="[8] \"Transfer File\": Value Change" {
          selector: _ -> [_ _ _ _ _ _ _ _ _ _ _ _ _ _ _]
          dyn-events: _ -> [_ _ _ _ _ _ _ _ _ _ _ _ _ _ _]
          timeout: 5 -> [_ _ _ _ _ _ _ _ _ _ _ _ _ _ _]
          tunnel: w175 -> [w439 _ _ _ _ _ _ _ _ _ _ _ _ _ _]
          tunnel: [w439 MegaAwesome_States."Re-Calculated Values" MegaAwesome_States."Calculated Values" MegaAwesome_States."Re-Calculated Values" MegaAwesome_States."Re-Calculated Values" MegaAwesome_States."Re-Calculated Values" MegaAwesome_States."Re-Calculated Values" MegaAwesome_States."Read Data" MegaAwesome_States."Read Data" MegaAwesome_States."No Event" MegaAwesome_States."No Event" MegaAwesome_States."No Event" MegaAwesome_States."No Event" MegaAwesome_States."No Event" MegaAwesome_States."No Event"] -> w174
          tunnel: w108 -> [w438 w440 w442 w444 w469 w497 w521 _ w550 w552 w565 w567 w571 w575 w579]
          tunnel: [w438 w440 w442 w444 w469 w497 w521 w540 w550 w552 w565 w567 w571 w575 w579] -> w167
          tunnel: w166 -> [_ _ _ _ _ _ _ w539 _ _ _ _ _ _ _]
          tunnel: w164 -> [_ _ _ _ _ _ _ _ _ _ _ _ _ _ _]
          event Timeout {
            n156 = event-data() -> ()  [unwired: 1 in, 2 out]
          }
          event "New: Dielectric", "New: Width", "New: Length", "New: Temp": Value Change {
            n157 = event-data() -> ()  [unwired: 1 in, 5 out]
          }
          event "Num Pts Log", "Transport Style Controls", "Num Pts": Value Change {
            n158 = event-data() -> ()  [unwired: 1 in, 5 out]
          }
          event "Sat-Trans Slider": Value Change {
            n159 = event-data() -> ()  [unwired: 1 in, 5 out]
            n160 = local read "Sqrt-Sat"() -> (w468:cluster{dbl[], dbl[]}[])
            n161 = Decimate 1D Array(w468) -> (w452:cluster{dbl[], dbl[]}[], w453:cluster{dbl[], dbl[]}[])
            n162 = local read "Slider Min"() -> (w449:dbl)
            n163 = local read "Sat-Trans Slider"() -> (w447:dbl)
            n164 = Array To Cluster(array=w452) -> (cluster=w467:T20)
            n165 = local read "New: Dielectric"() -> (w462:dbl)
            n166 = local read "Num Pts"() -> (w445:i32)
            n167 = local read "New: Width"() -> (w464:dbl)
            n168 = local read "New: Length"() -> (w463:dbl)
            n169 = Unbundle(w467) -> ("[0]"=w466:cluster{dbl[], dbl[]})  [unwired: 8 out]
            n170 = Absolute Value(x=w449) -> (abs(x)=w448:dbl)
            n171 = Unbundle(w466) -> (w450:dbl[], w465:dbl[])
            n172 = Add(x=w447, y=w448) -> (x+y=w446:dbl)
            n173 = Array Subset(array=w450, index=w446, length=w445) -> (w460:dbl[])
            n174 = local write "Sat Vg Array-Used"(w460) -> ()
            n175 = Array Subset(array=w465, index=w446, length=w445) -> (w461:dbl[])
            n176 = call "Mobility-Vt-Used Pts_Saturation.vi"("Width"=w464, "Length"=w463, "Dielectric (d)"=w462, "Sat Id Used"=w461, "Vg Used"=w460) -> ("Vt"=w456:dbl, "Mobility"=w457:dbl)  [unwired: 4 in, 1 out]
            n177 = local write "Index-Sat"(w446) -> ()
            n178 = local write "Sat Id-Used"(w461) -> ()
            n179 = Bundle(w460, w461) -> (w454:cluster{dbl[], dbl[]})  [unwired: 1 in]
            n180 = local read "Re-Calculated Values Cluster"() -> (w459:T9)
            n181 = Bundle By Name(cluster=w459, "Mobility-Sat"=w457, "Vt-Sat"=w456) -> (w458:T9)
            n182 = local write "Re-Calculated Values Cluster"(w458) -> ()
            n183 = Build Array (concatenate)(w452, w453, w454) -> (w451:cluster{dbl[], dbl[]}[])
            n184 = local write "Sqrt-Sat"(w451) -> ()
          }
          event "Lin-Trans Slider": Value Change {
            n185 = event-data() -> ()  [unwired: 1 in, 5 out]
            n186 = local read "Sqrt-Lin"() -> (w493:cluster{dbl[], dbl[]}[])
            n187 = Decimate 1D Array(w493) -> (w478:cluster{dbl[], dbl[]}[], w479:cluster{dbl[], dbl[]}[])
            n188 = local read "Slider Min"() -> (w475:dbl)
            n189 = Array To Cluster(array=w478) -> (cluster=w492:T20)
            n190 = local read "Lin-Trans Slider"() -> (w473:dbl)
            n191 = local read "New: Dielectric"() -> (w486:dbl)
            n192 = local read "Num Pts"() -> (w489:i32)
            n193 = local read "New: Width"() -> (w488:dbl)
            n194 = local read "New: Length"() -> (w487:dbl)
            n195 = local read "Lin Vd"() -> (w470:dbl)
            n196 = Unbundle(w492) -> ("[0]"=w491:cluster{dbl[], dbl[]})  [unwired: 8 out]
            n197 = Absolute Value(x=w475) -> (abs(x)=w474:dbl)
            n198 = Unbundle(w491) -> (w476:dbl[], w490:dbl[])
            n199 = Add(x=w473, y=w474) -> (x+y=w472:dbl)
            n200 = Array Subset(array=w476, index=w472, length=w489) -> (w484:dbl[])
            n201 = local write "Lin-Vg Array-Used"(w484) -> ()
            n202 = Array Subset(array=w490, index=w472, length=w489) -> (w485:dbl[])
            n203 = call "Mobility-Vt-Used Pts_Linear.vi"("Width"=w488, "Length"=w487, "Vd"=w470, "Dielectric (d)"=w486, "Id Used"=w485, "Vg Used"=w484) -> ("Mobility"=w481:dbl)  [unwired: 3 in, 2 out]
            n204 = local write "Index-Lin"(w472) -> ()
            n205 = local write "Lin Id-Used"(w485) -> ()
            n206 = Bundle(w484, w485) -> (w480:cluster{dbl[], dbl[]})  [unwired: 1 in]
            n207 = local read "Re-Calculated Values Cluster"() -> (w483:T9)
            n208 = Bundle By Name(cluster=w483, "Moblitity-Lin"=w481) -> (w482:T9)
            n209 = local write "Re-Calculated Values Cluster"(w482) -> ()
            n210 = Build Array (concatenate)(w478, w479, w480) -> (w477:cluster{dbl[], dbl[]}[])
            n211 = local write "Sqrt-Lin"(w477) -> ()
          }
          event "Sat-Log Slider": Value Change {
            n212 = event-data() -> ()  [unwired: 1 in, 5 out]
            n213 = local read "Sat-Log"() -> (w500:cluster{dbl[], dbl[]}[])
            n214 = Decimate 1D Array(w500) -> (w507:cluster{dbl[], dbl[]}[], w508:cluster{dbl[], dbl[]}[])
            n215 = local read "Slider Min"() -> (w504:dbl)
            n216 = Array To Cluster(array=w507) -> (cluster=w517:T20)
            n217 = property on="Sat-Log" class="XYGraph (strict)"("Active Plot"=u32 2, "Plot.Fill/Pt. Color"=u32 6618880, "Plot.Point Style"=u8 11) -> ()  [unwired: 2 in, 2 out]
            n218 = local read "Num Pts Log"() -> (w514:i32)
            n219 = local read "Sat-Log Slider"() -> (w502:dbl)
            n220 = Unbundle(w517) -> ("[0]"=w516:cluster{dbl[], dbl[]})  [unwired: 8 out]
            n221 = Absolute Value(x=w504) -> (abs(x)=w503:dbl)
            n222 = Unbundle(w516) -> (w505:dbl[], w515:dbl[])
            n223 = Add(x=w502, y=w503) -> (x+y=w499:dbl)
            n224 = Array Subset(array=w505, index=w499, length=w514) -> (w512:dbl[])
            n225 = Array Subset(array=w515, index=w499, length=w514) -> (w513:dbl[])
            n226 = local write "Vg Array-Log-Used"(w512) -> ()
            n227 = local write "IndexLog-Sat"(w499) -> ()
            n228 = Bundle(w512, w513) -> (w498:cluster{dbl[], dbl[]})  [unwired: 1 in]
            n229 = call "STS-Used.vi"("Id Used"=w513, "Vg-Used"=w512) -> ("STS"=w509:dbl)  [unwired: 9 in]
            n230 = local write "Sat Id-Log-Used"(w513) -> ()
            n231 = local read "Re-Calculated Values Cluster"() -> (w511:T9)
            n232 = Bundle By Name(cluster=w511, "STS"=w509) -> (w510:T9)
            n233 = local write "Re-Calculated Values Cluster"(w510) -> ()
            n234 = Build Array (concatenate)(w507, w508, w498) -> (w506:cluster{dbl[], dbl[]}[])
            n235 = local write "Sat-Log"(w506) -> ()
          }
          event "Lin-Log Slider": Value Change {
            n236 = event-data() -> ()  [unwired: 1 in, 5 out]
            n237 = local read "Lin-Log"() -> (w525:cluster{dbl[], dbl[]}[])
            n238 = Decimate 1D Array(w525) -> (w531:cluster{dbl[], dbl[]}[], w532:cluster{dbl[], dbl[]}[])
            n239 = local read "Slider Min"() -> (w528:dbl)
            n240 = Array To Cluster(array=w531) -> (cluster=w538:T20)
            n241 = local read "Num Pts Log"() -> (w535:i32)
            n242 = property on="Lin-Log" class="XYGraph (strict)"("Active Plot"=u32 2, "Plot.Fill/Pt. Color"=u32 6618880, "Plot.Point Style"=u8 11) -> ()  [unwired: 2 in, 2 out]
            n243 = local read "Lin-Log Slider"() -> (w526:dbl)
            n244 = Unbundle(w538) -> ("[0]"=w537:cluster{dbl[], dbl[]})  [unwired: 8 out]
            n245 = Absolute Value(x=w528) -> (abs(x)=w527:dbl)
            n246 = Unbundle(w537) -> (w529:dbl[], w536:dbl[])
            n247 = Add(x=w526, y=w527) -> (x+y=w524:dbl)
            n248 = Array Subset(array=w529, index=w524, length=w535) -> (w533:dbl[])
            n249 = local write "Lin-Vg Array-Log Used"(w533) -> ()
            n250 = Array Subset(array=w536, index=w524, length=w535) -> (w534:dbl[])
            n251 = local write "IndexLog-Sat"(w524) -> ()
            n252 = Bundle(w533, w534) -> (w523:cluster{dbl[], dbl[]})  [unwired: 1 in]
            n253 = local write "Lin Id-Log Used"(w534) -> ()
            n254 = Build Array (concatenate)(w531, w532, w523) -> (w530:cluster{dbl[], dbl[]}[])
            n255 = local write "Lin-Log"(w530) -> ()
          }
          event "Index Array": Value Change {
            n256 = event-data() -> ()  [unwired: 1 in, 5 out]
            n257 = Strip Path(path=w539) -> (stripped path=w545:path)  [unwired: 1 out]
            n258 = local write "Transfer Folder"(w545) -> ()
            n259 = List Folder(path=w545) -> (filenames=w541:string[])  [unwired: 3 in, 3 out]
            n260 = local read "Index Array"() -> (w540:i32)
            n261 = Path To String(path=w545) -> (string=w546:string)
            n262 = Index Array(array=w541, index=w540) -> (element=w547:string)
            n263 = Concatenate Strings(w546, "\\", w547) -> (w543:string)
            n264 = String To Path(string=w543) -> (path=w542:path)
            n265 = local write "Transfer File"(w542) -> ()
          }
          event "Transfer File": Value Change {
            w549 = path ""
            n266 = event-data() -> ()  [unwired: 1 in, 5 out]
            n267 = local write "Transport\nFolder"(w549) -> ()
            n268 = local write "Image Folder"(w549) -> ()
          }
          event "Remove Button": Mouse Down {
            w554 = 0
            n269 = event-data() -> ()  [unwired: 1 in, 5 out]
            n270 = property on="Image Out" class="ImageControl"() -> ("ROI"=w564:T18)  [unwired: 2 in, 2 out]
            n271 = Unbundle(w564) -> ("Global Rectangle"=w555:i32[], "Contours"=w557:T19)
            n272 = Reverse 1D Array(array=w555) -> (reversed array=w556:i32[])
            n273 = Reverse 1D Array(array=w557) -> (reversed array=w558:T19)
            n274 = Delete From Array(array=w556, index=w554) -> (array with subset deleted=w559:i32[])  [unwired: 1 in, 1 out]
            n275 = Delete From Array(array=w558, index=w554) -> (array with subset deleted=w560:T19)  [unwired: 1 in, 1 out]
            n276 = Reverse 1D Array(array=w559) -> (reversed array=w561:i32[])
            n277 = Reverse 1D Array(array=w560) -> (reversed array=w562:T19)
            n278 = Bundle(w561, w562) -> (w563:T21)  [unwired: 1 in]
            n279 = property on="Image Out" class="ImageControl"("ROI"=w563) -> ()  [unwired: 2 in, 2 out]
          }
          event "Undo Button": Mouse Down {
            n280 = event-data() -> ()  [unwired: 1 in, 5 out]
            n281 = invoke on="Image Out" class="ImageControl" method="Clear ROI"() -> ()  [unwired: 3 in, 3 out]
          }
          event "Image Folder": Value Change {
            n282 = event-data() -> ()  [unwired: 1 in, 5 out]
            n283 = local read "Image File"() -> (w569:path)
            n284 = call "Vision Acquisition"("Image Path"=w569) -> ("Image Out"=w570:T8)  [unwired: 25 in, 1 out]
            n285 = local write "Image Preview"(w570) -> ()
            n286 = local write "Image Out"(w570) -> ()
          }
          event "Zoom": Value Change {
            n287 = event-data() -> ()  [unwired: 1 in, 5 out]
            n288 = local read "Zoom"() -> (w574:i32)
            n289 = Bundle("Zoom"=w574, "Zoom"=w574) -> (w573:cluster{"Zoom":i32, "Zoom":i32})  [unwired: 1 in]
            n290 = property on="Image Out" class="ImageControl"("ZoomInteger"=w573) -> ()  [unwired: 2 in, 2 out]
          }
          event "Image Out": Mouse Enter {
            n291 = event-data() -> ()  [unwired: 1 in, 3 out]
            n292 = call "Simulate_Keyboard.vi"("Action"=u32 0, "Virtual Key"=u8 162) -> ()  [unwired: 7 in, 1 out]
          }
          event "Image Out": Mouse Leave {
            n293 = event-data() -> ()  [unwired: 1 in, 3 out]
            n294 = flat-sequence {
              frame #0 {
                n295 = Wait (ms)(milliseconds to wait=u32 10) -> ()  [unwired: 1 out]
              }
              frame #1 {
                n296 = call "Simulate_Keyboard.vi"("Action"=u32 2, "Virtual Key"=u8 162) -> ()  [unwired: 7 in, 1 out]
              }
            }
          }
        }
        n297 = Build Array(0.505025, 0.252522, 0.127742, 0.050345, 0.031129) -> (w131:dbl[])
        n298 = Array Subset(array=w131, index="Magnification", length=1) -> (w133:dbl[])
        n299 = To Double Precision Float(number=w133) -> (double precision float=w134:dbl[])
        n300 = for {
          N: w123 -> [_]
          shift-right: [w210] -> _
          shift-left: w122 -> [w210]
          shift-right: [w187] -> w110
          shift-left: w124 -> [w208]
          tunnel: w134 -> [w207]
          shift-right: [w204] -> _
          shift-left: w135 -> [w206]
          tunnel: w119 -> [w200]
          i -> [w203]
          n301 = Index Array(array=w210, index=w203) -> (element=w219:T22)
          n302 = Unbundle(w219) -> ("Points"=w218:i32[])  [unwired: 2 out]
          n303 = Array To Cluster(array=w218) -> (cluster=w217:T23)
          n304 = Unbundle(w217) -> ("Points[0]"=w199:i32, "Points[1]"=w186:i32, "Points[2]"=w209:i32, "Points[3]"=w215:i32)  [unwired: 5 out]
          n305 = Add(x=w199, y=10) -> (x+y=w197:i32)
          n306 = Subtract(x=w186, y=w215) -> (x-y=w214:i32)
          n307 = Subtract(x=w199, y=w209) -> (x-y=w216:i32)
          n308 = Square(x=w214) -> (x^2=w212:i32)
          n309 = Square(x=w216) -> (x^2=w213:i32)
          n310 = To Double Precision Float(number=w186) -> (double precision float=w185:dbl)
          n311 = Add(x=w213, y=w212) -> (x+y=w211:i32)
          n312 = Square Root(x=w211) -> (sqrt(x)=w191:dbl)
          n313 = Multiply(x=w191, y=0.5) -> (x*y=w194:dbl)
          n314 = Multiply(x=w191, y=w207) -> (x*y=w190:dbl[])
          n315 = Index Array(array=w190) -> (element=w202:dbl)  [unwired: 1 in]
          n316 = Number To Fractional String(number=w202, precision (6)=0) -> (F-format string=w201:string)  [unwired: 2 in]
          n317 = Build Array (concatenate)(w208, w190) -> (w188:dbl[])
          n318 = Add(x=w194, y=w185) -> (x+y=w196:dbl)
          n319 = Bundle(w197, w196) -> (w205:cluster{i32, dbl})  [unwired: 1 in]
          n320 = call "IMAQ Overlay Text"("BG Color (Transparent)"=u32 0, "Text Color (black)"=u32 16448250, "Font, Size & Style"=w200, "String"=w201, "Origin"=w205, "Image"=w206) -> ("Image Out"=w204:T8)  [unwired: 4 in, 1 out]
          n321 = To Long Integer(number=w188) -> (32bit integer=w187:i32[])
        }
        "Distances" <- w110
        n322 = Add Array Elements(numeric array=w110) -> (sum=w120:i32)
        n323 = local write "Total Width"(w120) -> ()
      }
      frame "Read Data" {
        n324 = call "IMAQ Dispose"("All Images? (No)"=TRUE) -> ()  [unwired: 5 in, 1 out]
        n325 = case shown="True" "Disable Flag" {
          tunnel: w630 -> [_ w655]
          tunnel: [w651 w652] -> w629
          tunnel: w627 -> [w651 _]
          frame False {
          }
          frame True {
            n326 = local read "Transfer Folder"() -> (w654:path)
            n327 = List Folder(path=w654) -> (filenames=w656:string[])  [unwired: 3 in, 3 out]
            n328 = Index Array(array=w656, index=w655) -> (element=w653:string)
            n329 = Build Path(base path=w654, name or relative path=w653) -> (appended path=w652:path)
            n330 = local write "Transfer File"(w652) -> ()
          }
        }
        n331 = call "Recorded Values.vi"("Path"=w629) -> ("Recorded Char"=→"Recorded Values Cluster":T9, "Recorded Prop"=w642:T1, "Fabrication Prop"=w640:T4)  [unwired: 8 in]
        n332 = Strip Path(path=w629) -> (stripped path=w639:path, name=w638:string)
        n333 = local write "Fabrication Prop"(w640) -> ()
        n334 = local write "Recorded Prop"(w642) -> ()
        n335 = Unbundle By Name(w642) -> ("Date Recorded"=→"Date Recorded":string, "Index"=w641:string, "Length"=w635:dbl, "Width"=w634:dbl)  [unwired: 1 out]
        n336 = Unbundle By Name(w642) -> ("Sample Temp"=w644:dbl)
        n337 = Unbundle By Name(w640) -> ("Dielectric (nm)"=w636:dbl, "Comments"=w637:string, "Date Created"=→"Date Created":string)
        n338 = List Folder(path=w639) -> (filenames=w633:string[])  [unwired: 3 in, 3 out]
        n339 = local write "Rec: Dielectric (d)"(w636) -> ()
        n340 = local write "Index"(w641) -> ()
        n341 = local write "Rec: Length"(w635) -> ()
        n342 = local write "Rec: Width"(w634) -> ()
        n343 = Equal To 0?(x=w644) -> (x = 0?=w647:bool)
        n344 = Number To Decimal String(number=w644) -> (decimal integer string=w648:string)  [unwired: 1 in]
        n345 = local write "Comments:"(w637) -> ()
        n346 = Search 1D Array(1D array=w633, element=w638) -> (index of element=w632:i32)  [unwired: 1 in]
        n347 = Equal?(x="", y=w648) -> (x = y?=w646:bool)
        n348 = Index Array(array=w633, index=w632) -> (element=→"Data Name:":string)
        n349 = local write "New: Width"(w634) -> ()
        n350 = local write "New: Length"(w635) -> ()
        n351 = local write "Index Array"(w632) -> ()
        n352 = Or(x=w647, y=w646) -> (x .or. y?=w645:bool)
        n353 = local write "New: Dielectric"(w636) -> ()
        n354 = case shown="True" w645 {
          tunnel: [w657 w658] -> w626
          tunnel: w644 -> [w657 _]
          frame False {
          }
          frame True {
            n355 = local read "Room Temp"() -> (w658:dbl)
          }
        }
        n356 = local write "New: Temp"(w626) -> ()
        n357 = Bundle By Name(cluster=w642, "Sample Temp"=w626) -> (w643:T1)
        n358 = local write "Rec: Temp"(w626) -> ()
        n359 = local write "Recorded Prop"(w643) -> ()
      }
      frame "Calculated Values" {
        n360 = local read "Image Center X"() -> (w660:i32)
        n361 = call "Image from TRF Display.vi"("Image Center X"=w660, "No Image File"=w705, "Image Folder"=w706, "Transfer File"=w675) -> ("Image Preview"=w667:T8, "Image Out"=w668:T8, "Image File"=w669:path, "Image Name"=→"Image Name":string, "ROI File"=w664:path)  [unwired: 3 in]
        n362 = invoke on="Image Out" class="ImageControl" method="Clear ROI"() -> ()  [unwired: 3 in, 3 out]
        n363 = local write "Image File"(w669) -> ()
        n364 = local write "Image Out"(w668) -> ()
        n365 = local write "Image Preview"(w667) -> ()
        n366 = call <vilib>:"Check if File or Folder Exists.vi"("path"=w664) -> ("file or folder exists?"=w665:bool, "dup path"=w666:path)  [unwired: 8 in, 1 out]
        n367 = case shown="True" w665 {
          tunnel: w666 -> [_ w726]
          frame False {
          }
          frame True {
            n368 = Read from Text File(file (use dialog)=w726) -> (text=w730:string)  [unwired: 3 in, 3 out]
            n369 = property on="Image Out" class="ImageControl"() -> ("ROI"=w727:T18)  [unwired: 2 in, 2 out]
            n370 = Unflatten From String(type=w727, binary string=w730) -> (value=w728:T18, error out=w729:errorcluster)  [unwired: 3 in, 1 out]
            n371 = property on="Image Out" class="ImageControl"(error in=w729, "ROI"=w728) -> ()  [unwired: 1 in, 2 out]
          }
        }
        n372 = call "TRF to TSP Plot_09_21_12a_JW.vi"("Transport Graph Properties"="Transport Style Controls", "No Transport File"=w670, "Transport Folder"=w671, "Transfer File"=w675) -> ("Transport"=w676:cluster{ext[], ext[]}[], "Transport File"=→"Transport\nFile":path, "Transport Name"=→"Transport Name:":string)  [unwired: 5 in]
        "Transport" <- w676
        n373 = Array Size(array=w676) -> (size(s)=w674:i32)
        n374 = local read "Image Center X"() -> (w661:i32)
        n375 = for {
          N: w674 -> [_]
          tunnel: "Transport Style Controls" -> [w734]
          i -> [w733]
          n376 = Unbundle By Name(w734) -> ("Transport Line Size"=w731:u16, "Transport Line Color"=w732:u32)
          n377 = property on="Transport" class="XYGraph (strict)"("Active Plot"=w733, "Plot.Plot Color"=w732, "Plot.Line Width"=w731) -> ()  [unwired: 2 in, 2 out]
        }
        n378 = local read "Recorded Prop"() -> (w708:T1)
        n379 = local read "Fabrication Prop"() -> (w715:T4)
        n380 = Bundle("Image Center X"=w661, 0) -> (w663:cluster{"Image Center X":i32, i32})  [unwired: 1 in]
        n381 = property on="Image Out" class="ImageControl"("Image Center Position"=w663) -> ()  [unwired: 2 in, 2 out]
        n382 = local read "Calculated Values Cluster"() -> (w725:T9)
        n383 = call "Mobility-Vt Calculator-File.vi"("NumPts"=w710, "Path"=w675) -> ("Used Points"=w703:T24, "Graph Cluster"=w693:T25, "Lin Vd"=w678:dbl, "Output"=w723:T26)  [unwired: 6 in]
        n384 = call "STS Calculator-File.vi"("NumPts"=w709, "Path"=w675) -> ("Used Points"=w698:T27, "XY Graph-Sat"=w682:cluster{dbl[], dbl[]}[], "XY Graph-Lin"=w679:cluster{dbl[], dbl[]}[], "Ouput"=w718:cluster{"STS-Sat":dbl, "STS-Lin":dbl})  [unwired: 6 in]
        n385 = Unbundle By Name(w715) -> ("Dielectric (nm)"=w713:dbl)
        n386 = Unbundle By Name(w708) -> ("Sample Temp"=w707:dbl)
        n387 = Unbundle By Name(w723) -> ("Mobility-Sat"=w722:dbl, "Vt-Sat"=w714:dbl, "Mobility-Lin"=w721:dbl, "Off I-Sat"=w720:dbl, "On/Off I-Sat"=w719:dbl)  [unwired: 1 out]
        n388 = local write "Lin Vd"(w678) -> ()
        n389 = Unbundle By Name(w718) -> ("STS-Sat"=w712:dbl)  [unwired: 1 out]
        n390 = local write "Sat-Log"(w682) -> ()
        n391 = local write "Lin-Log"(w679) -> ()
        n392 = call "Trap Density_VT.vi"("VT"=w714, "Dielectric"=w713) -> ("Trap Density-VT"=w717:dbl)
        n393 = call "Trap Density_STS.vi"("Temp (T) [K]"=w707, "S.T.S. (S)"=w712, "Dielectric"=w713) -> ("Trap Density (N)"=w716:dbl)  [unwired: 8 in]
        n394 = Bundle By Name(cluster=w725, "Mobility-Sat"=w722, "Moblitity-Lin"=w721, "On/Off"=w719, "Off Current"=w720, "Vt-Sat"=w714, "STS"=w712, "Trap Density-VT"=w717, "Trap Density-STS"=w716) -> (w724:T9)
        n395 = Unbundle By Name(w698) -> ("Sat Vg Used"=w697:dbl[], "Sat Log(Id) Used"=w696:dbl[], "Lin Vg Used"=w695:dbl[], "Lin Log(Id) Used"=w694:dbl[], "STS Index-Sat"=w680:dbl, "STS Index-Lin"=w681:dbl)
        n396 = Unbundle By Name(w703) -> ("Sat Vg Used"=w702:dbl[], "Sat Sqrt(Id) Used"=w701:dbl[], "Lin Vg Used"=w700:dbl[], "Lin Sqrt(Id) Used"=w699:dbl[], "Index-Lin"=w689:dbl, "Index-Sat"=w688:dbl)
        n397 = local write "Vg Array-Log-Used"(w697) -> ()
        n398 = local write "Sat Id-Log-Used"(w696) -> ()
        n399 = local write "Lin-Vg Array-Log Used"(w695) -> ()
        n400 = local write "Lin Id-Log Used"(w694) -> ()
        n401 = local write "IndexLog-Sat"(w680) -> ()
        n402 = local write "Index-Lin"(w681) -> ()
        n403 = local write "Calculated Values Cluster"(w724) -> ()
        n404 = local write "Sat Vg Array-Used"(w702) -> ()
        n405 = local write "Sat Id-Used"(w701) -> ()
        n406 = local write "Lin-Vg Array-Used"(w700) -> ()
        n407 = local write "Lin Id-Used"(w699) -> ()
        n408 = local write "Index-Sat"(w688) -> ()
        n409 = local write "Index-Lin"(w689) -> ()
        n410 = local write "Lin-Log Slider"(w681) -> ()
        n411 = local write "Sat-Log Slider"(w680) -> ()
        n412 = local write "Sat-Trans Slider"(w688) -> ()
        n413 = local write "Lin-Trans Slider"(w689) -> ()
        n414 = Unbundle By Name(w693) -> ("Raw Sat"=w687:cluster{dbl[], dbl[]}[], "Sqrt Sat"=w690:cluster{dbl[], dbl[]}[], "Raw Lin"=w692:cluster{dbl[], dbl[]}[], "Sqrt Lin"=w691:cluster{dbl[], dbl[]}[])
        n415 = Index Array(array=w687) -> (element=w686:cluster{dbl[], dbl[]})  [unwired: 1 in]
        n416 = Unbundle(w686) -> (w685:dbl[])  [unwired: 1 out]
        n417 = Array Max & Min(array=w685) -> (max value=w684:dbl, min value=w683:dbl)  [unwired: 2 out]
        n418 = property on="Sat-Trans Slider" class="Slide (strict)"("Scale.Maximum"=w684, "Scale.Minimum"=w683) -> ()  [unwired: 2 in, 2 out]
        n419 = property on="Lin-Trans Slider" class="Slide (strict)"("Scale.Maximum"=w684, "Scale.Minimum"=w683) -> ()  [unwired: 2 in, 2 out]
        n420 = property on="Sat-Log Slider" class="Slide (strict)"("Scale.Maximum"=w684, "Scale.Minimum"=w683) -> ()  [unwired: 2 in, 2 out]
        n421 = property on="Lin-Log Slider" class="Slide (strict)"("Scale.Maximum"=w684, "Scale.Minimum"=w683) -> ()  [unwired: 2 in, 2 out]
        n422 = local write "Slider Max"(w684) -> ()
        n423 = local write "Slider Min"(w683) -> ()
        n424 = local write "Raw- Sat"(w687) -> ()
        n425 = local write "Raw- Lin"(w692) -> ()
        n426 = local write "Sqrt-Sat"(w690) -> ()
        n427 = local write "Sqrt-Lin"(w691) -> ()
      }
      frame "Re-Calculated Values" {
        n428 = local read "Vg Array-Log-Used"() -> (w743:dbl[])
        n429 = local read "Sat Vg Array-Used"() -> (w751:dbl[])
        n430 = local read "Lin-Vg Array-Used"() -> (w757:dbl[])
        n431 = local read "Sat Id-Log-Used"() -> (w742:dbl[])
        n432 = local read "New: Dielectric"() -> (w755:dbl)
        n433 = local read "New: Dielectric"() -> (w740:dbl)
        n434 = local read "New: Length"() -> (w754:dbl)
        n435 = local read "New: Length"() -> (w750:dbl)
        n436 = local read "New: Width"() -> (w753:dbl)
        n437 = local read "New: Width"() -> (w749:dbl)
        n438 = local read "Lin Id-Used"() -> (w756:dbl[])
        n439 = local read "Sat Id-Used"() -> (w748:dbl[])
        n440 = local read "Re-Calculated Values Cluster"() -> (w759:T9)
        n441 = local read "New: Dielectric"() -> (w739:dbl)
        n442 = local read "New: Temp"() -> (w738:dbl)
        n443 = local read "Lin Vd"() -> (w735:dbl)
        n444 = call "Mobility-Vt-Used Pts_Saturation.vi"("Width"=w749, "Length"=w750, "Dielectric (d)"=w740, "Sat Id Used"=w748, "Vg Used"=w751) -> ("Vt"=w746:dbl, "Mobility"=w747:dbl)  [unwired: 4 in, 1 out]
        n445 = call "STS-Used.vi"("Id Used"=w742, "Vg-Used"=w743) -> ("STS"=w741:dbl)  [unwired: 9 in]
        n446 = call "Mobility-Vt-Used Pts_Linear.vi"("Width"=w753, "Length"=w754, "Vd"=w735, "Dielectric (d)"=w755, "Id Used"=w756, "Vg Used"=w757) -> ("Mobility"=w752:dbl)  [unwired: 3 in, 2 out]
        n447 = call "Trap Density_VT.vi"("VT"=w746, "Dielectric"=w740) -> ("Trap Density-VT"=w745:dbl)
        n448 = call "Trap Density_STS.vi"("Temp (T) [K]"=w738, "S.T.S. (S)"=w741, "Dielectric"=w739) -> ("Trap Density (N)"=w737:dbl)  [unwired: 8 in]
        n449 = Bundle By Name(cluster=w759, "Mobility-Sat"=w747, "Moblitity-Lin"=w752, "Vt-Sat"=w746, "STS"=w741, "Trap Density-VT"=w745, "Trap Density-STS"=w737) -> (w758:T9)
        n450 = local write "Re-Calculated Values Cluster"(w758) -> ()
      }
      frame "Next File" {
        n451 = call "IMAQ Dispose"("All Images? (No)"=TRUE) -> ()  [unwired: 5 in, 1 out]
        n452 = Strip Path(path=w776) -> (stripped path=w767:path, name=w774:string)
        n453 = local write "Transfer Folder"(w767) -> ()
        n454 = List Folder(path=w767) -> (filenames=w761:string[])  [unwired: 3 in, 3 out]
        n455 = Array Size(array=w761) -> (size(s)=w773:i32)
        n456 = Search 1D Array(1D array=w761, element=w774) -> (index of element=w771:i32)  [unwired: 1 in]
        n457 = Decrement(x=w773) -> (x-1=w772:i32)
        n458 = Equal?(x=w772, y=w771) -> (x = y?=w770:bool)
        n459 = case shown="True" w770 {
          tunnel: w763 -> [w778 _]
          tunnel: [w777 0] -> w762
          frame False {
            n460 = Increment(x=w778) -> (x+1=w777:i32)
          }
          frame True {
          }
        }
        n461 = Path To String(path=w767) -> (string=w768:string)
        n462 = Index Array(array=w761, index=w762) -> (element=w769:string)
        n463 = Concatenate Strings(w768, "\\", w769) -> (w765:string)
        n464 = String To Path(string=w765) -> (path=w764:path)
        n465 = local write "Transfer File"(w764) -> ()
      }
      frame "Previous File" {
        n466 = call "IMAQ Dispose"("All Images? (No)"=TRUE) -> ()  [unwired: 5 in, 1 out]
        n467 = Strip Path(path=w787) -> (stripped path=w784:path, name=w795:string)
        n468 = local write "Transfer Folder"(w784) -> ()
        n469 = List Folder(path=w784) -> (filenames=w788:string[])  [unwired: 3 in, 3 out]
        n470 = Array Size(array=w788) -> (size(s)=w782:i32)
        n471 = Search 1D Array(1D array=w788, element=w795) -> (index of element=w794:i32)  [unwired: 1 in]
        n472 = Decrement(x=w782) -> (x-1=w781:i32)
        n473 = Equal To 0?(x=w794) -> (x = 0?=w793:bool)
        n474 = case shown="True" w793 {
          tunnel: w786 -> [w798 _]
          tunnel: [w797 w799] -> w785
          tunnel: w781 -> [_ w799]
          frame False {
            n475 = Decrement(x=w798) -> (x-1=w797:i32)
          }
          frame True {
          }
        }
        n476 = Path To String(path=w784) -> (string=w783:string)
        n477 = Index Array(array=w788, index=w785) -> (element=w792:string)
        n478 = Concatenate Strings(w783, "\\", w792) -> (w790:string)
        n479 = String To Path(string=w790) -> (path=w789:path)
        n480 = local write "Transfer File"(w789) -> ()
      }
      frame "Discard File" {
        n481 = Strip Path(path=w814) -> (stripped path=w809:path, name=w808:string)
        n482 = property on="Disable Flag" class="Bool (strict)"("Value"=TRUE) -> ()  [unwired: 2 in, 2 out]
        n483 = List Folder(path=w809) -> (filenames=w807:string[])  [unwired: 3 in, 3 out]
        n484 = Search 1D Array(1D array=w807, element=w808) -> (index of element=w811:i32)  [unwired: 1 in]
        n485 = call "IMAQ Dispose"("All Images? (No)"=TRUE) -> ()  [unwired: 5 in, 1 out]
        n486 = Strip Path(path=w814) -> (stripped path=w806:path, name=w805:string)
        n487 = String Subset(string=w805, offset (0)=0, length (rest)=1) -> (substring=w802:string)
        n488 = Equal?(x=w802, y="X") -> (x = y?=w800:bool)
        n489 = case shown="False" w800 {
          tunnel: w806 -> [w822 _]
          tunnel: w814 -> [w818 _]
          tunnel: w805 -> [w817 _]
          tunnel: w811 -> [w816 w826]
          tunnel: [w816 w825] -> w810
          frame False {
            n490 = Path To String(path=w822) -> (string=w821:string)
            n491 = Concatenate Strings(w821, "\\", "X_", w817) -> (w820:string)
            n492 = String To Path(string=w820) -> (path=w819:path)
            n493 = Move(source path=w818, 10:w819) -> ()  [unwired: 3 in, 3 out]
          }
          frame True {
            n494 = Increment(x=w826) -> (x+1=w825:i32)
          }
        }
      }
      frame "Save" {
        n495 = stacked-sequence {
          seq-local: [w841 _] -> [_ w1315]
          seq-local: [w840 _] -> [_ w1313]
          tunnel: w833 -> [w842 w1316]
          frame #0 {
            # "Saves each Re-calculated parameter in sequence"
            n496 = stacked-sequence {
              tunnel: [_ _ _ _ _ _ _ _ _ _ _ _ _ w1285] -> w840
              tunnel: w842 -> [w862 _ _ _ _ _ _ _ _ _ _ _ _ _]
              frame #0 {
                n497 = call-poly <vilib>:"Read From Spreadsheet File.vi"("file path (dialog if empty)"=w862) -> ("all rows"=w861:string[][])  [unwired: 6 in, 4 out]
                n498 = Array Size(array=w861) -> (size(s)=w866:i32[])
                n499 = Array Subset(array=w861, index (row)=0, index (col)=0, length (col)=3) -> (w870:string[][])  [unwired: 1 in]
                n500 = Index Array(array=w866, index=0) -> (element=w864:i32)
                n501 = Reshape Array(w870, w864) -> (w863:string[])
                n502 = Search 1D Array(1D array=w863, element="Dielectric (nm):") -> (index of element=w873:i32)  [unwired: 1 in]
                n503 = Equal?(x=w873, y=-1) -> (x = y?=w872:bool)
                n504 = case shown="False" w872 {
                  tunnel: w861 -> [w880 w884]
                  tunnel: w873 -> [w878 _]
                  tunnel: [w877 w884] -> w871
                  frame False {
                    n505 = local read "Rec: Dielectric (d)"() -> (w882:dbl)
                    n506 = Number To Fractional String(number=w882) -> (F-format string=w879:string)  [unwired: 3 in]
                    n507 = Quotient & Remainder(x=w878, y=3) -> (floor(x/y)=w876:i32)  [unwired: 1 out]
                    n508 = Replace Array Subset(array=w880, new element=w879, index (row)=w876, index (col)=1) -> (w877:string[][])
                  }
                  frame True {
                  }
                }
                n509 = local write "Save Array"(w871) -> ()
              }
              frame #1 {
                n510 = local read "Save Array"() -> (w886:string[][])
                n511 = Array Size(array=w886) -> (size(s)=w889:i32[])
                n512 = Array Subset(array=w886, index (row)=0, index (col)=0, length (col)=3) -> (w893:string[][])  [unwired: 1 in]
                n513 = Index Array(array=w889, index=0) -> (element=w887:i32)
                n514 = Reshape Array(w893, w887) -> (w885:string[])
                n515 = Search 1D Array(1D array=w885, element="Comments:") -> (index of element=w896:i32)  [unwired: 1 in]
                n516 = Equal?(x=w896, y=-1) -> (x = y?=w895:bool)
                n517 = case shown="False" w895 {
                  tunnel: w886 -> [w904 w906]
                  tunnel: w896 -> [w901 _]
                  tunnel: [w903 w906] -> w894
                  frame False {
                    n518 = local read "Comments:"() -> (w902:string)
                    n519 = Quotient & Remainder(x=w901, y=3) -> (floor(x/y)=w899:i32)  [unwired: 1 out]
                    n520 = Replace Array Subset(array=w904, new element=w902, index (row)=w899, index (col)=1) -> (w903:string[][])
                  }
                  frame True {
                  }
                }
                n521 = local write "Save Array"(w894) -> ()
              }
              frame #2 {
                n522 = local read "Save Array"() -> (w908:string[][])
                n523 = Array Size(array=w908) -> (size(s)=w911:i32[])
                n524 = Array Subset(array=w908, index (row)=0, index (col)=0, length (col)=3) -> (w915:string[][])  [unwired: 1 in]
                n525 = Index Array(array=w911, index=0) -> (element=w909:i32)
                n526 = Reshape Array(w915, w909) -> (w907:string[])
                n527 = Search 1D Array(1D array=w907, element="Length (um):") -> (index of element=w918:i32)  [unwired: 1 in]
                n528 = Equal?(x=w918, y=-1) -> (x = y?=w917:bool)
                n529 = case shown="False" w917 {
                  tunnel: w908 -> [w927 w930]
                  tunnel: w918 -> [w926 _]
                  tunnel: [w925 w930] -> w916
                  frame False {
                    n530 = local read "New: Length"() -> (w922:dbl)
                    n531 = Quotient & Remainder(x=w926, y=3) -> (floor(x/y)=w921:i32)  [unwired: 1 out]
                    n532 = Format Value(format string="%#g", value (0)=w922) -> (output string=w923:string)  [unwired: 1 in]
                    n533 = Replace Array Subset(array=w927, new element=w923, index (row)=w921, index (col)=1) -> (w925:string[][])
                  }
                  frame True {
                  }
                }
                n534 = local write "Save Array"(w916) -> ()
              }
              frame #3 {
                n535 = local read "Save Array"() -> (w932:string[][])
                n536 = Array Size(array=w932) -> (size(s)=w937:i32[])
                n537 = Array Subset(array=w932, index (row)=0, index (col)=0, length (col)=3) -> (w933:string[][])  [unwired: 1 in]
                n538 = Index Array(array=w937, index=0) -> (element=w939:i32)
                n539 = Reshape Array(w933, w939) -> (w931:string[])
                n540 = Search 1D Array(1D array=w931, element="Width (um):") -> (index of element=w942:i32)  [unwired: 1 in]
                n541 = Equal?(x=w942, y=-1) -> (x = y?=w941:bool)
                n542 = case shown="False" w941 {
                  tunnel: w942 -> [w951 _]
                  tunnel: w932 -> [w950 w954]
                  tunnel: [w949 w954] -> w940
                  frame False {
                    n543 = local read "New: Width"() -> (w946:dbl)
                    n544 = Quotient & Remainder(x=w951, y=3) -> (floor(x/y)=w945:i32)  [unwired: 1 out]
                    n545 = Format Value(format string="%#g", value (0)=w946) -> (output string=w947:string)  [unwired: 1 in]
                    n546 = Replace Array Subset(array=w950, new element=w947, index (row)=w945, index (col)=1) -> (w949:string[][])
                  }
                  frame True {
                  }
                }
                n547 = local write "Save Array"(w940) -> ()
              }
              frame #4 {
                w964 = "Sample Temp (K):"
                n548 = local read "Save Array"() -> (w956:string[][])
                n549 = Array Size(array=w956) -> (size(s)=w961:i32[])
                n550 = Array Subset(array=w956, index (row)=0, index (col)=0, length (col)=3) -> (w957:string[][])  [unwired: 1 in]
                n551 = Index Array(array=w961, index=0) -> (element=w963:i32)
                n552 = Reshape Array(w957, w963) -> (w955:string[])
                n553 = Search 1D Array(1D array=w955, element=w964) -> (index of element=w967:i32)  [unwired: 1 in]
                n554 = Equal?(x=w967, y=-1) -> (x = y?=w966:bool)
                n555 = case shown="False" w966 {
                  tunnel: w956 -> [w975 w988]
                  tunnel: w967 -> [w974 _]
                  tunnel: [w973 w987] -> w965
                  tunnel: w955 -> [_ w990]
                  tunnel: w964 -> [_ w979]
                  frame False {
                    n556 = local read "New: Temp"() -> (w971:dbl)
                    n557 = Quotient & Remainder(x=w974, y=3) -> (floor(x/y)=w969:i32)  [unwired: 1 out]
                    n558 = Format Value(format string="%#g", value (0)=w971) -> (output string=w970:string)  [unwired: 1 in]
                    n559 = Replace Array Subset(array=w975, new element=w970, index (row)=w969, index (col)=1) -> (w973:string[][])
                  }
                  frame True {
                    n560 = local read "New: Temp"() -> (w981:dbl)
                    n561 = Search 1D Array(1D array=w990, element="Width (um):") -> (index of element=w985:i32)  [unwired: 1 in]
                    n562 = Quotient & Remainder(x=w985, y=3) -> (floor(x/y)=w978:i32)  [unwired: 1 out]
                    n563 = Increment(x=w978) -> (x+1=w984:i32)
                    n564 = Format Value(format string="%#g", value (0)=w981) -> (output string=w980:string)  [unwired: 1 in]
                    n565 = Build Array(w979, w980) -> (w983:string[])
                    n566 = Insert Into Array(array=w988, index (row)=w984, new element=w983) -> (w987:string[][])  [unwired: 1 in]
                  }
                }
                n567 = local write "Save Array"(w965) -> ()
              }
              frame #5 {
                w1000 = "Mobility-Sat (cm^2/Vs):"
                n568 = local read "Save Array"() -> (w992:string[][])
                n569 = Array Size(array=w992) -> (size(s)=w997:i32[])
                n570 = Array Subset(array=w992, index (row)=0, index (col)=0, length (col)=3) -> (w993:string[][])  [unwired: 1 in]
                n571 = Index Array(array=w997, index=0) -> (element=w999:i32)
                n572 = Reshape Array(w993, w999) -> (w991:string[])
                n573 = Search 1D Array(1D array=w991, element=w1000) -> (index of element=w1003:i32)  [unwired: 1 in]
                n574 = Equal?(x=w1003, y=-1) -> (x = y?=w1002:bool)
                n575 = case shown="False" w1002 {
                  tunnel: w992 -> [w1012 w1022]
                  tunnel: w1003 -> [w1011 _]
                  tunnel: [w1010 w1021] -> w1001
                  tunnel: w991 -> [_ w1019]
                  tunnel: w1000 -> [_ w1018]
                  frame False {
                    n576 = local read "Re-Calculated Values Cluster"() -> (w1007:T9)
                    n577 = Unbundle By Name(w1007) -> ("Mobility-Sat"=w1006:dbl)
                    n578 = Quotient & Remainder(x=w1011, y=3) -> (floor(x/y)=w1005:i32)  [unwired: 1 out]
                    n579 = Format Value(format string="%#g", value (0)=w1006) -> (output string=w1008:string)  [unwired: 1 in]
                    n580 = Replace Array Subset(array=w1012, new element=w1008, index (row)=w1005, index (col)=1) -> (w1010:string[][])
                  }
                  frame True {
                    n581 = local read "Re-Calculated Values Cluster"() -> (w1017:T9)
                    n582 = Unbundle By Name(w1017) -> ("Mobility-Sat"=w1016:dbl)
                    n583 = Search 1D Array(1D array=w1019, element="Mobility (cm^2/Vs):") -> (index of element=w1025:i32)  [unwired: 1 in]
                    n584 = Quotient & Remainder(x=w1025, y=3) -> (floor(x/y)=w1015:i32)  [unwired: 1 out]
                    n585 = Format Value(format string="%#g", value (0)=w1016) -> (output string=w1020:string)  [unwired: 1 in]
                    n586 = Build Array(w1018, w1020) -> (w1024:string[])
                    n587 = Replace Array Subset(array=w1022, new element=w1024, index (row)=w1015) -> (w1021:string[][])  [unwired: 1 in]
                  }
                }
                n588 = local write "Save Array"(w1001) -> ()
              }
              frame #6 {
                w1037 = "Mobility-Lin (cm^2/Vs):"
                n589 = local read "Save Array"() -> (w1028:string[][])
                n590 = Array Size(array=w1028) -> (size(s)=w1034:i32[])
                n591 = Array Subset(array=w1028, index (row)=0, index (col)=0, length (col)=3) -> (w1030:string[][])  [unwired: 1 in]
                n592 = Index Array(array=w1034, index=0) -> (element=w1036:i32)
                n593 = Reshape Array(w1030, w1036) -> (w1029:string[])
                n594 = Search 1D Array(1D array=w1029, element=w1037) -> (index of element=w1040:i32)  [unwired: 1 in]
                n595 = Equal?(x=w1040, y=-1) -> (x = y?=w1039:bool)
                n596 = case shown="True" w1039 {
                  tunnel: w1028 -> [w1049 w1058]
                  tunnel: w1040 -> [w1048 _]
                  tunnel: [w1047 w1057] -> w1038
                  tunnel: w1029 -> [_ w1056]
                  tunnel: w1037 -> [_ w1055]
                  frame False {
                    n597 = local read "Re-Calculated Values Cluster"() -> (w1044:T9)
                    n598 = Unbundle By Name(w1044) -> ("Moblitity-Lin"=w1043:dbl)
                    n599 = Quotient & Remainder(x=w1048, y=3) -> (floor(x/y)=w1042:i32)  [unwired: 1 out]
                    n600 = Format Value(format string="%#g", value (0)=w1043) -> (output string=w1045:string)  [unwired: 1 in]
                    n601 = Replace Array Subset(array=w1049, new element=w1045, index (row)=w1042, index (col)=1) -> (w1047:string[][])
                  }
                  frame True {
                    n602 = local read "Re-Calculated Values Cluster"() -> (w1054:T9)
                    n603 = Unbundle By Name(w1054) -> ("Moblitity-Lin"=w1053:dbl)
                    n604 = Search 1D Array(1D array=w1056, element="Mobility-Sat (cm^2/Vs):") -> (index of element=w1062:i32)  [unwired: 1 in]
                    n605 = Quotient & Remainder(x=w1062, y=3) -> (floor(x/y)=w1052:i32)  [unwired: 1 out]
                    n606 = Format Value(format string="%#g", value (0)=w1053) -> (output string=w1065:string)  [unwired: 1 in]
                    n607 = Build Array(w1055, w1065) -> (w1060:string[])
                    n608 = Increment(x=w1052) -> (x+1=w1061:i32)
                    n609 = Insert Into Array(array=w1058, index (row)=w1061, new element=w1060) -> (w1057:string[][])  [unwired: 1 in]
                  }
                }
                n610 = local write "Save Array"(w1038) -> ()
              }
              frame #7 {
                w1075 = "On/Off I-Sat:"
                n611 = local read "Save Array"() -> (w1066:string[][])
                n612 = Array Size(array=w1066) -> (size(s)=w1072:i32[])
                n613 = Array Subset(array=w1066, index (row)=0, index (col)=0, length (col)=3) -> (w1068:string[][])  [unwired: 1 in]
                n614 = Index Array(array=w1072, index=0) -> (element=w1074:i32)
                n615 = Reshape Array(w1068, w1074) -> (w1067:string[])
                n616 = Search 1D Array(1D array=w1067, element=w1075) -> (index of element=w1078:i32)  [unwired: 1 in]
                n617 = Equal?(x=w1078, y=-1) -> (x = y?=w1077:bool)
                n618 = case shown="True" w1077 {
                  tunnel: w1066 -> [w1087 w1096]
                  tunnel: w1078 -> [w1086 _]
                  tunnel: [w1085 w1097] -> w1076
                  tunnel: w1067 -> [_ w1094]
                  tunnel: w1075 -> [_ w1093]
                  frame False {
                    n619 = local read "Calculated Values Cluster"() -> (w1082:T9)
                    n620 = Quotient & Remainder(x=w1086, y=3) -> (floor(x/y)=w1080:i32)  [unwired: 1 out]
                    n621 = Unbundle By Name(w1082) -> ("On/Off"=w1081:dbl)
                    n622 = Format Value(format string="%#g", value (0)=w1081) -> (output string=w1083:string)  [unwired: 1 in]
                    n623 = Replace Array Subset(array=w1087, new element=w1083, index (row)=w1080, index (col)=1) -> (w1085:string[][])
                  }
                  frame True {
                    n624 = local read "Calculated Values Cluster"() -> (w1092:T9)
                    n625 = Unbundle By Name(w1092) -> ("On/Off"=w1091:dbl)
                    n626 = Search 1D Array(1D array=w1094, element="On/Off Current:") -> (index of element=w1100:i32)  [unwired: 1 in]
                    n627 = Quotient & Remainder(x=w1100, y=3) -> (floor(x/y)=w1090:i32)  [unwired: 1 out]
                    n628 = Format Value(format string="%#g", value (0)=w1091) -> (output string=w1095:string)  [unwired: 1 in]
                    n629 = Build Array(w1093, w1095) -> (w1099:string[])
                    n630 = Replace Array Subset(array=w1096, new element=w1099, index (row)=w1090) -> (w1097:string[][])  [unwired: 1 in]
                  }
                }
                n631 = local write "Save Array"(w1076) -> ()
              }
              frame #8 {
                w1112 = "Off I-Sat (A):"
                n632 = local read "Save Array"() -> (w1103:string[][])
                n633 = Array Size(array=w1103) -> (size(s)=w1109:i32[])
                n634 = Array Subset(array=w1103, index (row)=0, index (col)=0, length (col)=3) -> (w1105:string[][])  [unwired: 1 in]
                n635 = Index Array(array=w1109, index=0) -> (element=w1111:i32)
                n636 = Reshape Array(w1105, w1111) -> (w1104:string[])
                n637 = Search 1D Array(1D array=w1104, element=w1112) -> (index of element=w1115:i32)  [unwired: 1 in]
                n638 = Equal?(x=w1115, y=-1) -> (x = y?=w1114:bool)
                n639 = case shown="True" w1114 {
                  tunnel: w1103 -> [w1124 w1133]
                  tunnel: w1115 -> [w1123 _]
                  tunnel: [w1122 w1132] -> w1113
                  tunnel: w1104 -> [_ w1131]
                  tunnel: w1112 -> [_ w1130]
                  frame False {
                    # "New Data File"
                    n640 = local read "Calculated Values Cluster"() -> (w1119:T9)
                    n641 = Unbundle By Name(w1119) -> ("Off Current"=w1118:dbl)
                    n642 = Quotient & Remainder(x=w1123, y=3) -> (floor(x/y)=w1117:i32)  [unwired: 1 out]
                    n643 = Format Value(format string="%#g", value (0)=w1118) -> (output string=w1120:string)  [unwired: 1 in]
                    n644 = Replace Array Subset(array=w1124, new element=w1120, index (row)=w1117, index (col)=1) -> (w1122:string[][])
                  }
                  frame True {
                    # "Old Data File"
                    n645 = local read "Calculated Values Cluster"() -> (w1129:T9)
                    n646 = Unbundle By Name(w1129) -> ("Off Current"=w1128:dbl)
                    n647 = Search 1D Array(1D array=w1131, element="On/Off I-Sat:") -> (index of element=w1137:i32)  [unwired: 1 in]
                    n648 = Quotient & Remainder(x=w1137, y=3) -> (floor(x/y)=w1127:i32)  [unwired: 1 out]
                    n649 = Format Value(format string="%#g", value (0)=w1128) -> (output string=w1140:string)  [unwired: 1 in]
                    n650 = Build Array(w1130, w1140) -> (w1135:string[])
                    n651 = Increment(x=w1127) -> (x+1=w1136:i32)
                    n652 = Insert Into Array(array=w1133, index (row)=w1136, new element=w1135) -> (w1132:string[][])  [unwired: 1 in]
                  }
                }
                n653 = local write "Save Array"(w1113) -> ()
              }
              frame #9 {
                w1142 = "Vt-Sat (V):"
                n654 = local read "Save Array"() -> (w1143:string[][])
                n655 = Array Size(array=w1143) -> (size(s)=w1148:i32[])
                n656 = Array Subset(array=w1143, index (row)=0, index (col)=0, length (col)=3) -> (w1144:string[][])  [unwired: 1 in]
                n657 = Index Array(array=w1148, index=0) -> (element=w1150:i32)
                n658 = Reshape Array(w1144, w1150) -> (w1141:string[])
                n659 = Search 1D Array(1D array=w1141, element=w1142) -> (index of element=w1153:i32)  [unwired: 1 in]
                n660 = Equal?(x=w1153, y=-1) -> (x = y?=w1152:bool)
                n661 = case shown="False" w1152 {
                  tunnel: w1143 -> [w1161 w1171]
                  tunnel: w1153 -> [w1159 _]
                  tunnel: [w1158 w1170] -> w1151
                  tunnel: w1142 -> [_ w1169]
                  tunnel: w1141 -> [_ w1168]
                  frame False {
                    n662 = local read "Re-Calculated Values Cluster"() -> (w1157:T9)
                    n663 = Unbundle By Name(w1157) -> ("Vt-Sat"=w1156:dbl)
                    n664 = Quotient & Remainder(x=w1159, y=3) -> (floor(x/y)=w1155:i32)  [unwired: 1 out]
                    n665 = Number To Fractional String(number=w1156) -> (F-format string=w1160:string)  [unwired: 3 in]
                    n666 = Replace Array Subset(array=w1161, new element=w1160, index (row)=w1155, index (col)=1) -> (w1158:string[][])
                  }
                  frame True {
                    n667 = local read "Re-Calculated Values Cluster"() -> (w1166:T9)
                    n668 = Unbundle By Name(w1166) -> ("Vt-Sat"=w1165:dbl)
                    n669 = Search 1D Array(1D array=w1168, element="Threshold V (V):") -> (index of element=w1167:i32)  [unwired: 1 in]
                    n670 = Quotient & Remainder(x=w1167, y=3) -> (floor(x/y)=w1164:i32)  [unwired: 1 out]
                    n671 = Format Value(format string="%#g", value (0)=w1165) -> (output string=w1176:string)  [unwired: 1 in]
                    n672 = Build Array(w1169, w1176) -> (w1173:string[])
                    n673 = Replace Array Subset(array=w1171, new element=w1173, index (row)=w1164) -> (w1170:string[][])  [unwired: 1 in]
                  }
                }
                n674 = local write "Save Array"(w1151) -> ()
              }
              frame #10 {
                n675 = disable-structure shown="Disabled" {
                  frame Disabled {
                    n676 = local read "Save Array"() -> (w1177:string[][])
                    n677 = Array Size(array=w1177) -> (size(s)=w1183:i32[])
                    n678 = Array Subset(array=w1177, index (row)=0, index (col)=0, length (col)=3) -> (w1179:string[][])  [unwired: 1 in]
                    n679 = Index Array(array=w1183, index=0) -> (element=w1185:i32)
                    n680 = Reshape Array(w1179, w1185) -> (w1178:string[])
                    n681 = Search 1D Array(1D array=w1178, element="VT-Lin (V):") -> (index of element=w1188:i32)  [unwired: 1 in]
                    n682 = Equal?(x=w1188, y=-1) -> (x = y?=w1187:bool)
                    n683 = case shown="True" w1187 {
                      tunnel: w1177 -> [w1196 w1199]
                      tunnel: w1188 -> [w1195 _]
                      tunnel: [w1194 w1199] -> w1186
                      frame False {
                        n684 = Quotient & Remainder(x=w1195, y=3) -> (floor(x/y)=w1191:i32)  [unwired: 1 out]
                        n685 = Format Value(format string="%#g") -> (output string=w1192:string)  [unwired: 2 in]
                        n686 = Replace Array Subset(array=w1196, new element=w1192, index (row)=w1191, index (col)=1) -> (w1194:string[][])
                      }
                      frame True {
                      }
                    }
                    n687 = local write "Save Array"(w1186) -> ()
                  }
                  frame Enabled {
                  }
                }
              }
              frame #11 {
                w1200 = "STS-Sat (V/decade):"
                n688 = local read "Save Array"() -> (w1202:string[][])
                n689 = Array Size(array=w1202) -> (size(s)=w1207:i32[])
                n690 = Array Subset(array=w1202, index (row)=0, index (col)=0, length (col)=3) -> (w1203:string[][])  [unwired: 1 in]
                n691 = Index Array(array=w1207, index=0) -> (element=w1209:i32)
                n692 = Reshape Array(w1203, w1209) -> (w1201:string[])
                n693 = Search 1D Array(1D array=w1201, element=w1200) -> (index of element=w1212:i32)  [unwired: 1 in]
                n694 = Equal?(x=w1212, y=-1) -> (x = y?=w1211:bool)
                n695 = case shown="True" w1211 {
                  tunnel: w1202 -> [w1221 w1229]
                  tunnel: w1212 -> [w1220 _]
                  tunnel: [w1219 w1230] -> w1210
                  tunnel: w1201 -> [_ w1228]
                  tunnel: w1200 -> [_ w1227]
                  frame False {
                    # "Current Data File"
                    n696 = local read "Re-Calculated Values Cluster"() -> (w1215:T9)
                    n697 = Unbundle By Name(w1215) -> ("STS"=w1216:dbl)
                    n698 = Quotient & Remainder(x=w1220, y=3) -> (floor(x/y)=w1214:i32)  [unwired: 1 out]
                    n699 = Format Value(format string="%#g", value (0)=w1216) -> (output string=w1217:string)  [unwired: 1 in]
                    n700 = Replace Array Subset(array=w1221, new element=w1217, index (row)=w1214, index (col)=1) -> (w1219:string[][])
                  }
                  frame True {
                    # "Old Data File"
                    n701 = local read "Re-Calculated Values Cluster"() -> (w1225:T9)
                    n702 = Unbundle By Name(w1225) -> ("STS"=w1226:dbl)
                    n703 = Search 1D Array(1D array=w1228, element="S.T.S. (V/decade):") -> (index of element=w1233:i32)  [unwired: 1 in]
                    n704 = Quotient & Remainder(x=w1233, y=3) -> (floor(x/y)=w1224:i32)  [unwired: 1 out]
                    n705 = Format Value(format string="%#g", value (0)=w1226) -> (output string=w1236:string)  [unwired: 1 in]
                    n706 = Build Array(w1227, w1236) -> (w1232:string[])
                    n707 = Replace Array Subset(array=w1229, new element=w1232, index (row)=w1224) -> (w1230:string[][])  [unwired: 1 in]
                  }
                }
                n708 = local write "Save Array"(w1210) -> ()
              }
              frame #12 {
                w1237 = "Trap Density-VT (Traps/Vcm^2):"
                n709 = local read "Save Array"() -> (w1239:string[][])
                n710 = Array Size(array=w1239) -> (size(s)=w1244:i32[])
                n711 = Array Subset(array=w1239, index (row)=0, index (col)=0, length (col)=3) -> (w1240:string[][])  [unwired: 1 in]
                n712 = Index Array(array=w1244, index=0) -> (element=w1246:i32)
                n713 = Reshape Array(w1240, w1246) -> (w1238:string[])
                n714 = Search 1D Array(1D array=w1238, element=w1237) -> (index of element=w1249:i32)  [unwired: 1 in]
                n715 = Equal?(x=w1249, y=-1) -> (x = y?=w1248:bool)
                n716 = case shown="True" w1248 {
                  tunnel: w1239 -> [w1258 w1266]
                  tunnel: w1249 -> [w1256 _]
                  tunnel: [w1255 w1267] -> w1247
                  tunnel: w1238 -> [_ w1265]
                  tunnel: w1237 -> [_ w1264]
                  frame False {
                    n717 = local read "Re-Calculated Values Cluster"() -> (w1253:T9)
                    n718 = Unbundle By Name(w1253) -> ("Trap Density-VT"=w1252:dbl)
                    n719 = Quotient & Remainder(x=w1256, y=3) -> (floor(x/y)=w1251:i32)  [unwired: 1 out]
                    n720 = Format Value(format string="%#g", value (0)=w1252) -> (output string=w1257:string)  [unwired: 1 in]
                    n721 = Replace Array Subset(array=w1258, new element=w1257, index (row)=w1251, index (col)=1) -> (w1255:string[][])
                  }
                  frame True {
                    n722 = local read "Re-Calculated Values Cluster"() -> (w1263:T9)
                    n723 = Unbundle By Name(w1263) -> ("Trap Density-VT"=w1262:dbl)
                    n724 = Search 1D Array(1D array=w1265, element="STS-Sat (V/decade):") -> (index of element=w1271:i32)  [unwired: 1 in]
                    n725 = Quotient & Remainder(x=w1271, y=3) -> (floor(x/y)=w1261:i32)  [unwired: 1 out]
                    n726 = Format Value(format string="%#g", value (0)=w1262) -> (output string=w1268:string)  [unwired: 1 in]
                    n727 = Build Array(w1264, w1268) -> (w1273:string[])
                    n728 = Increment(x=w1261) -> (x+1=w1272:i32)
                    n729 = Insert Into Array(array=w1266, index (row)=w1272, new element=w1273) -> (w1267:string[][])  [unwired: 1 in]
                  }
                }
                n730 = local write "Save Array"(w1247) -> ()
              }
              frame #13 {
                w1275 = "Trap Density-STS (Traps/Vcm^2):"
                n731 = local read "Save Array"() -> (w1277:string[][])
                n732 = Array Size(array=w1277) -> (size(s)=w1282:i32[])
                n733 = Array Subset(array=w1277, index (row)=0, index (col)=0, length (col)=3) -> (w1278:string[][])  [unwired: 1 in]
                n734 = Index Array(array=w1282, index=0) -> (element=w1284:i32)
                n735 = Reshape Array(w1278, w1284) -> (w1276:string[])
                n736 = Search 1D Array(1D array=w1276, element=w1275) -> (index of element=w1287:i32)  [unwired: 1 in]
                n737 = Equal?(x=w1287, y=-1) -> (x = y?=w1286:bool)
                n738 = case shown="False" w1286 {
                  tunnel: w1277 -> [w1296 w1304]
                  tunnel: w1287 -> [w1295 _]
                  tunnel: [w1294 w1305] -> w1285
                  tunnel: w1276 -> [_ w1303]
                  tunnel: w1275 -> [_ w1302]
                  frame False {
                    n739 = local read "Re-Calculated Values Cluster"() -> (w1291:T9)
                    n740 = Unbundle By Name(w1291) -> ("Trap Density-STS"=w1290:dbl)
                    n741 = Quotient & Remainder(x=w1295, y=3) -> (floor(x/y)=w1289:i32)  [unwired: 1 out]
                    n742 = Format Value(format string="%#g", value (0)=w1290) -> (output string=w1292:string)  [unwired: 1 in]
                    n743 = Replace Array Subset(array=w1296, new element=w1292, index (row)=w1289, index (col)=1) -> (w1294:string[][])
                  }
                  frame True {
                    n744 = local read "Re-Calculated Values Cluster"() -> (w1301:T9)
                    n745 = Unbundle By Name(w1301) -> ("Trap Density-STS"=w1300:dbl)
                    n746 = Search 1D Array(1D array=w1303, element="Trap Density-VT (Traps/Vcm^2):") -> (index of element=w1309:i32)  [unwired: 1 in]
                    n747 = Quotient & Remainder(x=w1309, y=3) -> (floor(x/y)=w1299:i32)  [unwired: 1 out]
                    n748 = Format Value(format string="%#g", value (0)=w1300) -> (output string=w1312:string)  [unwired: 1 in]
                    n749 = Build Array(w1302, w1312) -> (w1307:string[])
                    n750 = Increment(x=w1299) -> (x+1=w1308:i32)
                    n751 = Insert Into Array(array=w1304, index (row)=w1308, new element=w1307) -> (w1305:string[][])  [unwired: 1 in]
                  }
                }
                n752 = local write "Save Array"(w1285) -> ()
              }
            }
            n753 = local read "New: Temp"() -> (w843:dbl)
            n754 = local read "New: Width"() -> (w844:dbl)
            n755 = local read "New: Length"() -> (w846:dbl)
            n756 = local read "Index"() -> (w845:string)
            n757 = To Long Integer(number=w843) -> (32bit integer=w860:i32)
            n758 = Number To Decimal String(number=w860) -> (decimal integer string=w855:string)  [unwired: 1 in]
            n759 = To Long Integer(number=w844) -> (32bit integer=w859:i32)
            n760 = To Long Integer(number=w846) -> (32bit integer=w858:i32)
            n761 = Strip Path(path=w842) -> (stripped path=w847:path)  [unwired: 1 out]
            n762 = Number To Decimal String(number=w858) -> (decimal integer string=w853:string)  [unwired: 1 in]
            n763 = Number To Decimal String(number=w859) -> (decimal integer string=w852:string)  [unwired: 1 in]
            n764 = Concatenate Strings("_", w855, "K") -> (w857:string)
            n765 = call "Build Text"("Temp"=w857, "Index"=w845, "Length"=w853, "Width"=w852) -> ("Result"=w851:string)  [unwired: 10 in, 1 out]
            n766 = Path To String(path=w847) -> (string=w849:string)
            n767 = Concatenate Strings(w849, "\\", w851) -> (w850:string)
            n768 = String To Path(string=w850) -> (path=w841:path)
          }
          frame #1 {
            n769 = flat-sequence {
              tunnel: w1316 -> [w1318]
              tunnel: w1315 -> [w1317]
              tunnel: [w1317] -> w1314
              tunnel: w1314 -> [w1324]
              tunnel: w1313 -> [w1323]
              frame #0 {
                n770 = Equal?(x=w1318, y=w1317) -> (x = y?=w1319:bool)
                n771 = case shown="False" w1319 {
                  tunnel: w1318 -> [w1322 _]
                  tunnel: w1317 -> [w1321 _]
                  frame False {
                    n772 = Move(source path=w1322, 9:TRUE, 10:w1321) -> ()  [unwired: 2 in, 3 out]
                  }
                  frame True {
                  }
                }
              }
              frame #1 {
                n773 = local write "Transfer File"(w1324) -> ()
                n774 = call-poly <vilib>:"Write To Spreadsheet File.vi"("2D data"=w1323, "file path (dialog if empty)"=w1324) -> ()  [unwired: 6 in, 1 out]
              }
            }
          }
        }
        n775 = local read "Save Next?"() -> (w827:bool)
        n776 = Cluster To Array(cluster=w832) -> (array=w831:bool[])
        n777 = Boolean Array To Number(Boolean array=w831) -> (number=w830:u32)
        n778 = Equal To 0?(x=w830) -> (x = 0?=w829:bool)
        n779 = case shown="True" w829 {
          tunnel: [MegaAwesome_States."Read Data" w839] -> w828
          tunnel: w827 -> [_ w836]
          frame False {
          }
          frame True {
            n780 = Select(t=MegaAwesome_States."Next File", s=w836, f=MegaAwesome_States."No Event") -> (s? t:f=w839:T2)
          }
        }
      }
      frame "Exit" {
        n781 = disable-structure shown="Disabled" {
          disable-tunnel: [w1328 _] -> _
          disable-tunnel: [w1327 _] -> _
          frame Disabled {
            n782 = flat-sequence {
              tunnel: [w1337] -> w1328
              tunnel: [w1337] -> w1327
              frame #0 {
                w1336 = FALSE
                n783 = property on="Next File" class="Bool (strict)"("Value"=w1336) -> (error out=w1331:errorcluster)  [unwired: 2 in, 1 out]
                n784 = property on="Previous File" class="Bool (strict)"(error in=w1331, "Value"=w1336) -> (error out=w1332:errorcluster)  [unwired: 1 in, 1 out]
                n785 = Request Deallocation(TRUE) -> ()
                n786 = property on="Save" class="Bool (strict)"(error in=w1332, "Value"=w1336) -> (error out=w1333:errorcluster)  [unwired: 1 in, 1 out]
                n787 = property on="Export" class="Bool (strict)"("Value"=w1336) -> ()  [unwired: 2 in, 2 out]
                n788 = property on="Save Next" class="Bool (strict)"(error in=w1333, "Value"=w1336) -> (error out=w1334:errorcluster)  [unwired: 1 in, 1 out]
                n789 = property on="Discard" class="Bool (strict)"(error in=w1334, "Value"=w1336) -> (error out=w1335:errorcluster)  [unwired: 1 in, 1 out]
                n790 = property on="Save Lines" class="Bool (strict)"(error in=w1335, "Value"=w1336) -> ()  [unwired: 1 in, 2 out]
                n791 = property on="Close" class="Bool (strict)"("Value"=w1336) -> ()  [unwired: 2 in, 2 out]
                n792 = property on="Disable Flag" class="Bool (strict)"("Value"=w1336) -> ()  [unwired: 2 in, 2 out]
                n793 = call "IMAQ Dispose"("All Images? (No)"=TRUE) -> ()  [unwired: 5 in, 1 out]
              }
              frame #1 {
                w1337 = MegaAwesome_States."Exit"
              }
            }
          }
          frame Enabled {
          }
        }
        n794 = event shown="[0] Application Instance Close?" {
          selector: _ -> [_]
          dyn-events: _ -> [_]
          timeout: _ -> [_]
          event Application Instance Close? {
            n795 = event-data() -> ()  [unwired: 1 in, 4 out]
            n796 = event-data("Discard?"=TRUE) -> ()  [unwired: 2 in, 1 out]
          }
        }
      }
      frame "Save Lines" {
        n797 = Build Path(base path=w1340, name or relative path="ROI") -> (appended path=w1343:path)
        n798 = call <vilib>:"Check if File or Folder Exists.vi"("path"=w1343) -> ("file or folder exists?"=w1341:bool, "dup path"=w1344:path)  [unwired: 8 in, 1 out]
        n799 = case shown="False" w1341 {
          tunnel: w1344 -> [w1352 w1353]
          tunnel: [w1351 w1353] -> w1348
          frame False {
            n800 = Create Folder(path (use dialog)=w1352) -> (created path=w1351:path)  [unwired: 2 in, 2 out]
          }
          frame True {
          }
        }
        n801 = local read "Index"() -> (w1339:string)
        n802 = property on="Image Out" class="ImageControl"() -> ("ROI"=w1345:T18)  [unwired: 2 in, 2 out]
        n803 = Build Path(base path=w1348, name or relative path=w1339) -> (appended path=w1347:path)
        n804 = Flatten To String(anything=w1345) -> (data string=w1346:string)  [unwired: 3 in, 2 out]
        n805 = Write to Text File(file (use dialog)=w1347, text=w1346) -> ()  [unwired: 2 in, 3 out]
      }
      frame "Export" {
        n806 = flat-sequence {
          tunnel: ["Independant Variable:"] -> w1354
          tunnel: w1355 -> [w1411]
          tunnel: w1354 -> [w1410]
          frame #0 {
            n807 = stacked-sequence {
              tunnel: "Independant Variable:" -> [w1359 w1364 w1369 w1374 w1379 w1384 w1389 w1394 w1399 w1404]
              frame #0 {
                n808 = Equal?(x=w1359, y="Length (um):") -> (x = y?=w1360:bool)
                n809 = case shown="True" w1360 {
                  frame False {
                  }
                  frame True {
                    n810 = local write "X Axis Display Type"("1") -> ()
                    n811 = local write "Opj X Axis"("2") -> ()
                  }
                }
              }
              frame #1 {
                n812 = Equal?(x=w1364, y="Sample Temp (K):") -> (x = y?=w1365:bool)
                n813 = case shown="True" w1365 {
                  frame False {
                  }
                  frame True {
                    n814 = local write "X Axis Display Type"("1") -> ()
                    n815 = local write "Opj X Axis"("1") -> ()
                  }
                }
              }
              frame #2 {
                n816 = Equal?(x=w1369, y="Mobility-Sat (cm^2/Vs):") -> (x = y?=w1370:bool)
                n817 = case shown="True" w1370 {
                  frame False {
                  }
                  frame True {
                    n818 = local write "X Axis Display Type"("2") -> ()
                    n819 = local write "Opj X Axis"("2") -> ()
                  }
                }
              }
              frame #3 {
                n820 = Equal?(x=w1374, y="Mobility-Lin (cm^2/Vs):") -> (x = y?=w1375:bool)
                n821 = case shown="True" w1375 {
                  frame False {
                  }
                  frame True {
                    n822 = local write "X Axis Display Type"("2") -> ()
                    n823 = local write "Opj X Axis"("2") -> ()
                  }
                }
              }
              frame #4 {
                n824 = Equal?(x=w1379, y="On/Off I-Sat:") -> (x = y?=w1380:bool)
                n825 = case shown="True" w1380 {
                  frame False {
                  }
                  frame True {
                    n826 = local write "X Axis Display Type"("2") -> ()
                    n827 = local write "Opj X Axis"("2") -> ()
                  }
                }
              }
              frame #5 {
                n828 = Equal?(x=w1384, y="Off I-Sat (A):") -> (x = y?=w1385:bool)
                n829 = case shown="True" w1385 {
                  frame False {
                  }
                  frame True {
                    n830 = local write "X Axis Display Type"("2") -> ()
                    n831 = local write "Opj X Axis"("2") -> ()
                  }
                }
              }
              frame #6 {
                n832 = Equal?(x=w1389, y="Vt-Sat (V):") -> (x = y?=w1390:bool)
                n833 = case shown="True" w1390 {
                  frame False {
                  }
                  frame True {
                    n834 = local write "X Axis Display Type"("1") -> ()
                    n835 = local write "Opj X Axis"("1") -> ()
                  }
                }
              }
              frame #7 {
                n836 = Equal?(x=w1394, y="STS-Sat (V/decade):") -> (x = y?=w1395:bool)
                n837 = case shown="True" w1395 {
                  frame False {
                  }
                  frame True {
                    n838 = local write "Opj X Axis"("1") -> ()
                    n839 = local write "X Axis Display Type"("1") -> ()
                  }
                }
              }
              frame #8 {
                n840 = Equal?(x=w1399, y="Trap Density-VT (Traps/Vcm^2):") -> (x = y?=w1400:bool)
                n841 = case shown="True" w1400 {
                  frame False {
                  }
                  frame True {
                    n842 = local write "X Axis Display Type"("2") -> ()
                    n843 = local write "Opj X Axis"("2") -> ()
                  }
                }
              }
              frame #9 {
                n844 = Equal?(x=w1404, y="Trap Density-STS (Traps/Vcm^2):") -> (x = y?=w1405:bool)
                n845 = case shown="True" w1405 {
                  frame False {
                  }
                  frame True {
                    n846 = local write "X Axis Display Type"("2") -> ()
                    n847 = local write "Opj X Axis"("2") -> ()
                  }
                }
              }
            }
          }
          frame #1 {
            n848 = local read "Transfer Folder"() -> (w1415:path)
            n849 = Build Path(base path=w1415, name or relative path="Stats") -> (appended path=w1416:path)
            n850 = call <vilib>:"Check if File or Folder Exists.vi"("path"=w1416) -> ("file or folder exists?"=w1430:bool, "dup path"=w1429:path)  [unwired: 8 in, 1 out]
            n851 = call "OA_ConnectToOrigin.vi"() -> ("error out"=w1427:errorcluster, "Origin.IOApplication"=w1428:refnum<k7>)  [unwired: 8 in]
            n852 = case shown="False" w1430 {
              tunnel: w1429 -> [w1603 w1604]
              tunnel: [w1602 w1604] -> w1414
              frame False {
                n853 = Create Folder(path (use dialog)=w1603) -> (created path=w1602:path)  [unwired: 2 in, 2 out]
              }
              frame True {
              }
            }
            n854 = call "File Dialog"("start path"=w1416) -> ("selected path"=w1418:path)  [unwired: 11 in, 3 out]
            n855 = call "OA_Load.vi"("error in (no error)"=w1427, "Path"=w1411, "Origin.IOApplication"=w1428) -> ("error out"=w1425:errorcluster, "Origin.IOApplication"=w1426:refnum<k7>)  [unwired: 1 out]
            n856 = call "OAExecute.vi"("script"="document -m 3;", "Error IO"=w1425, "Origin.IOApplication"=w1426) -> ("Error IO Out"=w1423:errorcluster, "Origin.IOApplication"=w1424:refnum<k7>)  [unwired: 1 in, 1 out]
            n857 = stacked-sequence {
              tunnel: w1415 -> [w1441 w1471 w1483 w1505 w1525 w1546 w1567 w1590]
              tunnel: w1414 -> [w1442 w1470 w1484 w1504 w1526 w1547 w1568 w1591]
              tunnel: w1424 -> [w1444 w1468 w1486 w1507 w1528 w1549 w1570 w1593]
              tunnel: w1423 -> [w1443 w1469 w1485 w1506 w1527 w1548 w1569 w1592]
              tunnel: [_ _ _ _ _ _ _ w1588] -> w1413
              tunnel: [_ _ _ _ _ _ _ w1589] -> w1412
              tunnel: w1410 -> [w1440 w1461 w1482 w1503 w1524 w1545 w1566 w1587]
              frame #0 {
                n858 = local read "X Axis Display Type"() -> (w1432:string)
                n859 = local read "Opj X Axis"() -> (w1437:string)
                n860 = Concatenate Strings("window -a MOBLGraph;\nlayer.x.type=", w1437, "; layer.x.label.numFormat = ", w1432, "; Y3 = 1; X3 = 1;", "window -a MOBLTable;\nwindow -s TV;") -> (w1435:string)
                n861 = call "Param_Analysis_7_24b_JW.vi"("Independant Variable"=w1440, "error in (no error)"=w1443, "Data Folder"=w1441, "Parameter String"="Mobility-Lin (cm^2/Vs):", "Parameter Name"="Mobility-Lin", "Stats Folder"=w1442) -> ("error out"=w1446:errorcluster, "Output Array"=w1448:string[][], "Variables"=w1439:T28)  [unwired: 2 in, 1 out]
                n862 = call "Origin_Export_7_27a_JW.vi"("Input Conditions"=w1439, "Analysis Array"=w1448, "error in (no error)"=w1446, "Parameter Worksheet Name"="[MOBLTable]Mobilities", "Parameter Folder Script"="pe_cd \"Mobility-Lin\";", "Origin.IOApplication"=w1444) -> ("error out"=w1445:errorcluster, "reference out"=w1447:refnum<k7>)  [unwired: 3 in, 1 out]
                n863 = call "OAExecute.vi"("script"=w1435, "Error IO"=w1445, "Origin.IOApplication"=w1447) -> ()  [unwired: 1 in, 3 out]
              }
              frame #1 {
                n864 = local read "X Axis Display Type"() -> (w1453:string)
                n865 = local read "Opj X Axis"() -> (w1458:string)
                n866 = Concatenate Strings("window -a MOBSGraph;\nlayer.x.type=", w1458, "; layer.x.label.numFormat = ", w1453, "; Y3 = 1; X3 = 1;", "window -a MOBSTable;\nwindow -s TV;") -> (w1456:string)
                n867 = call "Param_Analysis_7_24b_JW.vi"("Independant Variable"=w1461, "error in (no error)"=w1469, "Data Folder"=w1471, "Parameter String"="Mobility-Sat (cm^2/Vs):", "Parameter Name"="Mobility-Sat", "Stats Folder"=w1470) -> ("error out"=w1464:errorcluster, "Output Array"=w1462:string[][], "Variables"=w1460:T28)  [unwired: 2 in, 1 out]
                n868 = call "Origin_Export_7_27a_JW.vi"("Input Conditions"=w1460, "Analysis Array"=w1462, "error in (no error)"=w1464, "Parameter Worksheet Name"="[MOBSTable]Mobilities", "Parameter Folder Script"="pe_cd \"Mobility-Sat\";", "Origin.IOApplication"=w1468) -> ("error out"=w1463:errorcluster, "reference out"=w1465:refnum<k7>)  [unwired: 3 in, 1 out]
                n869 = call "OAExecute.vi"("script"=w1456, "Error IO"=w1463, "Origin.IOApplication"=w1465) -> ()  [unwired: 1 in, 3 out]
              }
              frame #2 {
                n870 = local read "X Axis Display Type"() -> (w1474:string)
                n871 = local read "Opj X Axis"() -> (w1479:string)
                n872 = Concatenate Strings("window -a NSTSGraph;\nlayer.x.type=", w1479, "; layer.x.label.numFormat = ", w1474, "; Y3 = 1; X3 = 1;", "window -a NSTSTable;\nwindow -s TV;") -> (w1477:string)
                n873 = call "Param_Analysis_7_24b_JW.vi"("Independant Variable"=w1482, "error in (no error)"=w1485, "Data Folder"=w1483, "Parameter String"="Trap Density-STS (Traps/Vcm^2):", "Parameter Name"="Trap Density-STS", "Stats Folder"=w1484) -> ("error out"=w1489:errorcluster, "Output Array"=w1487:string[][], "Variables"=w1481:T28)  [unwired: 2 in, 1 out]
                n874 = call "Origin_Export_7_27a_JW.vi"("Input Conditions"=w1481, "Analysis Array"=w1487, "error in (no error)"=w1489, "Parameter Worksheet Name"="[NSTSTable]Trap Densities", "Parameter Folder Script"="pe_cd \"N-STS\";", "Origin.IOApplication"=w1486) -> ("error out"=w1488:errorcluster, "reference out"=w1490:refnum<k7>)  [unwired: 3 in, 1 out]
                n875 = call "OAExecute.vi"("script"=w1477, "Error IO"=w1488, "Origin.IOApplication"=w1490) -> ()  [unwired: 1 in, 3 out]
              }
              frame #3 {
                n876 = local read "X Axis Display Type"() -> (w1495:string)
                n877 = local read "Opj X Axis"() -> (w1500:string)
                n878 = call "Param_Analysis_7_24b_JW.vi"("Independant Variable"=w1503, "error in (no error)"=w1506, "Data Folder"=w1505, "Parameter String"="Trap Density-VT (Traps/Vcm^2):", "Parameter Name"="Trap Density-Vt", "Stats Folder"=w1504) -> ("error out"=w1510:errorcluster, "Output Array"=w1508:string[][], "Variables"=w1502:T28)  [unwired: 2 in, 1 out]
                n879 = Concatenate Strings("window -a NVtGraph;\nlayer.x.type=", w1500, "; layer.x.label.numFormat = ", w1495, "; Y3 = 1; X3 = 1;", "window -a NVtTable;\nwindow -s TV;") -> (w1498:string)
                n880 = call "Origin_Export_7_27a_JW.vi"("Input Conditions"=w1502, "Analysis Array"=w1508, "error in (no error)"=w1510, "Parameter Worksheet Name"="[NVTTable]Trap Densities", "Parameter Folder Script"="pe_cd \"N-Vt\";", "Origin.IOApplication"=w1507) -> ("error out"=w1509:errorcluster, "reference out"=w1511:refnum<k7>)  [unwired: 3 in, 1 out]
                n881 = call "OAExecute.vi"("script"=w1498, "Error IO"=w1509, "Origin.IOApplication"=w1511) -> ()  [unwired: 1 in, 3 out]
              }
              frame #4 {
                n882 = local read "X Axis Display Type"() -> (w1516:string)
                n883 = local read "Opj X Axis"() -> (w1521:string)
                n884 = Concatenate Strings("window -a OffIGraph;\nlayer.x.type=", w1521, "; layer.x.label.numFormat = ", w1516, "; Y3 = 1; X3 = 1;", "window -a OffITable;\nwindow -s TV;") -> (w1519:string)
                n885 = call "Param_Analysis_7_24b_JW.vi"("Independant Variable"=w1524, "error in (no error)"=w1527, "Data Folder"=w1525, "Parameter String"="Off I-Sat (A):", "Parameter Name"="Off I-Sat", "Stats Folder"=w1526) -> ("error out"=w1531:errorcluster, "Output Array"=w1529:string[][], "Variables"=w1523:T28)  [unwired: 2 in, 1 out]
                n886 = call "Origin_Export_7_27a_JW.vi"("Input Conditions"=w1523, "Analysis Array"=w1529, "error in (no error)"=w1531, "Parameter Worksheet Name"="[OffItable]OffCurrents", "Parameter Folder Script"="pe_cd \"OffI-Sat\";", "Origin.IOApplication"=w1528) -> ("error out"=w1530:errorcluster, "reference out"=w1532:refnum<k7>)  [unwired: 3 in, 1 out]
                n887 = call "OAExecute.vi"("script"=w1519, "Error IO"=w1530, "Origin.IOApplication"=w1532) -> ()  [unwired: 1 in, 3 out]
              }
              frame #5 {
                n888 = local read "X Axis Display Type"() -> (w1537:string)
                n889 = local read "Opj X Axis"() -> (w1542:string)
                n890 = Concatenate Strings("window -a OnOffGraph;\nlayer.x.type=", w1542, "; layer.x.label.numFormat = ", w1537, "; Y3 = 1; X3 = 1;", "window -a OnOffTable;\nwindow -s TV;") -> (w1540:string)
                n891 = call "Param_Analysis_7_24b_JW.vi"("Independant Variable"=w1545, "error in (no error)"=w1548, "Data Folder"=w1546, "Parameter String"="On/Off I-Sat:", "Parameter Name"="OnOff Ratio", "Stats Folder"=w1547) -> ("error out"=w1552:errorcluster, "Output Array"=w1550:string[][], "Variables"=w1544:T28)  [unwired: 2 in, 1 out]
                n892 = call "Origin_Export_7_27a_JW.vi"("Input Conditions"=w1544, "Analysis Array"=w1550, "error in (no error)"=w1552, "Parameter Worksheet Name"="[OnOffTable]On/Off Ratios", "Parameter Folder Script"="pe_cd \"OnOff-Ratio\";", "Origin.IOApplication"=w1549) -> ("error out"=w1551:errorcluster, "reference out"=w1553:refnum<k7>)  [unwired: 3 in, 1 out]
                n893 = call "OAExecute.vi"("script"=w1540, "Error IO"=w1551, "Origin.IOApplication"=w1553) -> ()  [unwired: 1 in, 3 out]
              }
              frame #6 {
                n894 = local read "X Axis Display Type"() -> (w1558:string)
                n895 = local read "Opj X Axis"() -> (w1563:string)
                n896 = call "Param_Analysis_7_24b_JW.vi"("Independant Variable"=w1566, "error in (no error)"=w1569, "Data Folder"=w1567, "Parameter String"="STS-Sat (V/decade):", "Parameter Name"="STS-Sat", "Stats Folder"=w1568) -> ("error out"=w1573:errorcluster, "Output Array"=w1571:string[][], "Variables"=w1565:T28)  [unwired: 2 in, 1 out]
                n897 = Concatenate Strings("window -a SGraph;\nlayer.x.type=", w1563, "; layer.x.label.numFormat = ", w1558, "; Y3 = 1; X3 = 1;", "window -a STable;\nwindow -s TV;") -> (w1561:string)
                n898 = call "Origin_Export_7_27a_JW.vi"("Input Conditions"=w1565, "Analysis Array"=w1571, "error in (no error)"=w1573, "Parameter Worksheet Name"="[STable]Threshold Swing", "Parameter Folder Script"="pe_cd \"STS-Sat\";", "Origin.IOApplication"=w1570) -> ("error out"=w1572:errorcluster, "reference out"=w1574:refnum<k7>)  [unwired: 3 in, 1 out]
                n899 = call "OAExecute.vi"("script"=w1561, "Error IO"=w1572, "Origin.IOApplication"=w1574) -> ()  [unwired: 1 in, 3 out]
              }
              frame #7 {
                n900 = local read "X Axis Display Type"() -> (w1579:string)
                n901 = local read "Opj X Axis"() -> (w1584:string)
                n902 = Concatenate Strings("window -a VtGraph;\nlayer.x.type=", w1584, "; layer.x.label.numFormat = ", w1579, "; Y3 = 1; X3 = 1;", "window -a VtTable;\nwindow -s TV;") -> (w1582:string)
                n903 = call "Param_Analysis_7_24b_JW.vi"("Independant Variable"=w1587, "error in (no error)"=w1592, "Data Folder"=w1590, "Parameter String"="Vt-Sat (V):", "Parameter Name"="Vt-Sat", "Stats Folder"=w1591) -> ("error out"=w1596:errorcluster, "Output Array"=w1594:string[][], "Variables"=w1586:T28)  [unwired: 2 in, 1 out]
                n904 = call "Origin_Export_7_27a_JW.vi"("Input Conditions"=w1586, "Analysis Array"=w1594, "error in (no error)"=w1596, "Parameter Worksheet Name"="[VtTable]Threshold Voltages", "Parameter Folder Script"="pe_cd \"Vt-Sat\";", "Origin.IOApplication"=w1593) -> ("error out"=w1595:errorcluster, "reference out"=w1597:refnum<k7>)  [unwired: 3 in, 1 out]
                n905 = call "OAExecute.vi"("script"=w1582, "Error IO"=w1595, "Origin.IOApplication"=w1597) -> ("Error IO Out"=w1588:errorcluster, "Origin.IOApplication"=w1589:refnum<k7>)  [unwired: 1 in, 1 out]
              }
            }
            n906 = Path To String(path=w1418) -> (string=w1417:string)
            n907 = call "OAExecute.vi"("script"="pe_cd /; ", "Error IO"=w1413, "Origin.IOApplication"=w1412) -> ("Error IO Out"=w1419:errorcluster, "Origin.IOApplication"=w1420:refnum<k7>)  [unwired: 1 in, 1 out]
            n908 = call "OASaveProject.vi"("path"=w1417, "Error IO"=w1419, "Origin.IOApplication"=w1420) -> ("Origin.IOApplication"=w1409:refnum<k7>)  [unwired: 2 out]
            n909 = call "OAEndSession.vi"("Origin.IOApplication"=w1409) -> ()  [unwired: 1 in, 3 out]
          }
        }
      }
    }
    "Current State" <- w11
    "Folder Index" <- w21
    n910 = Wait (ms)(milliseconds to wait=u32 50) -> ()  [unwired: 1 out]
    n911 = Equal?(x=w11, y=MegaAwesome_States."Exit") -> (x = y?=w14:bool)
  }
  n912 = disable-structure shown="Disabled" {
    disable-tunnel: w1 -> [w1606 _]
    frame Disabled {
      n913 = call "Close LabView?"("Enable"=w1606) -> ("OK"=w1605:bool)  [unwired: 17 in, 1 out]
      n914 = Quit LabVIEW(quit? (T)=w1605) -> ()
    }
    frame Enabled {
    }
  }
